vi "GDSIconEditor_CreateVIIcon.vi"(6 "ViRef(IgnoreIfNotWired)":refnum<vi>, 7 "AutomaticUpdateNoQuestionsAsked(False)":bool, 8 "error in (no error)":errorcluster, 9 "Application:Menu Launch:VI":string, 10 "Application:Menu Launch:App":refnum<vi>) -> (0 "error out":errorcluster)   [LabVIEW 2016]
uses:
  <resource>/Framework/Providers/Open_GDS/ClassProviders/Common/LvIcon_class/GDSLvIcon_ColorControl.ctl
  <resource>/Framework/Providers/Open_GDS/SubVIs/GOOP_HelpButton.ctl
  <resource>/Framework/Providers/Open_GDS/ClassProviders/Common/IconEditor/private/GDSIconEditor_ScopeType.ctl
  <vilib>/picture/picture.llb/imagedata.ctl
  <vilib>/Utility/miscctls.llb/LVPoint32TypeDef.ctl
  <resource>/Framework/Providers/Open_GDS/ClassProviders/Provider_LvNativeClass/ClassWriterNative_class/IconSize.ctl
  <resource>/Framework/Providers/Open_GDS/ClassProviders/Common/LvIcon_class/subvis/GDSLvIcon_TextDataType.ctl
  <resource>/Framework/Providers/Open_GDS/ClassProviders/Common/LvIcon_class/GDSLvIcon_WordCompressionType.ctl
  <resource>/Framework/Providers/Open_GDS/ClassProviders/Common/LvIcon_class/GDSLvIcon_TextAlignment.ctl
  <vilib>/Utility/miscctls.llb/LVRectTypeDef.ctl
  <vilib>/Utility/miscctls.llb/LVPositionTypeDef.ctl
  <vilib>/event_ctls.llb/lveventtype.ctl
  <vilib>/Utility/miscctls.llb/LVPointTypeDef.ctl
  <resource>/Framework/Providers/Open_GDS/ClassProviders/Provider_LvNativeClass/ClassWriterNative_class/ClassWriterNative.lvclass
  <vilib>/Utility/cursorutil.llb/Set Cursor (Icon Pict).vi
panel:
  in  "_HideHeader":bool=TRUE caption="Force Capital Letters"
  out "_IconPreview":picture caption="Icon Preview"
  out "DragIcon":picture
  in  "_MethodIconName":string caption="Body Text"
  in  "FloodFillMask":bool
  out "_IconName":string
  in  "_IconSearchText":string caption="Icon search text"
  in  "_Manage":bool
  in  "_Folders":u16(ring) caption="Folders" items=["<All icons>", "...EW 2014\\resource\\Framework\\Providers\\Icons", "...source\\Framework\\Providers\\Open_GDS\\Glyphs", "...esource\\Framework\\Providers\\Open_GDS\\Icons"]
  out "Icons":picture
  in  "_Icons":bool
  in  "_TextAlignment":u16(ring) caption="Text Alignment" items=["Center", "Left", "Right"]
  in  "_IconSize":u16(ring) caption="Icon Size" items=["Full", "1 c-term high", "2 c-term high", "3 c-term high", "4 c-term high"]
  in  "_HelpCreateViIcon":T1
  out "_FilePrefixFound":string caption="Prefix found"
  in  "_ApplyHeaderToAll":bool caption="Apply this header to all\nVIs/Ctrls in this folder"
  in  "_BodyTextColor":T2 caption="Body Text"
  in  "_BackgroundColor":T2 caption="Body Background"
  in  "_FontCompression":enum16{"Auto", "On", "Off"}(ring) caption="Font Compression"
  in  "_FontCapitalOnly":bool=TRUE caption="Force Capital Letters"
  out "_After":picture caption="New"
  out "_ViNotSavedMessage":string caption="VI not saved. Please select a path!"
  in  "Cancel":bool
  in  "Accept":bool
  in  "_EditHeader":bool
  in  "_TemplateVI":bool
  in  "_VIPath":path caption="VI Path"
  out "_Before":picture caption="Current"
  out "_Scope":string caption="Visibility"
  in  "Icon not available":picture
  in  "_OCR":bool
  # "Icon"
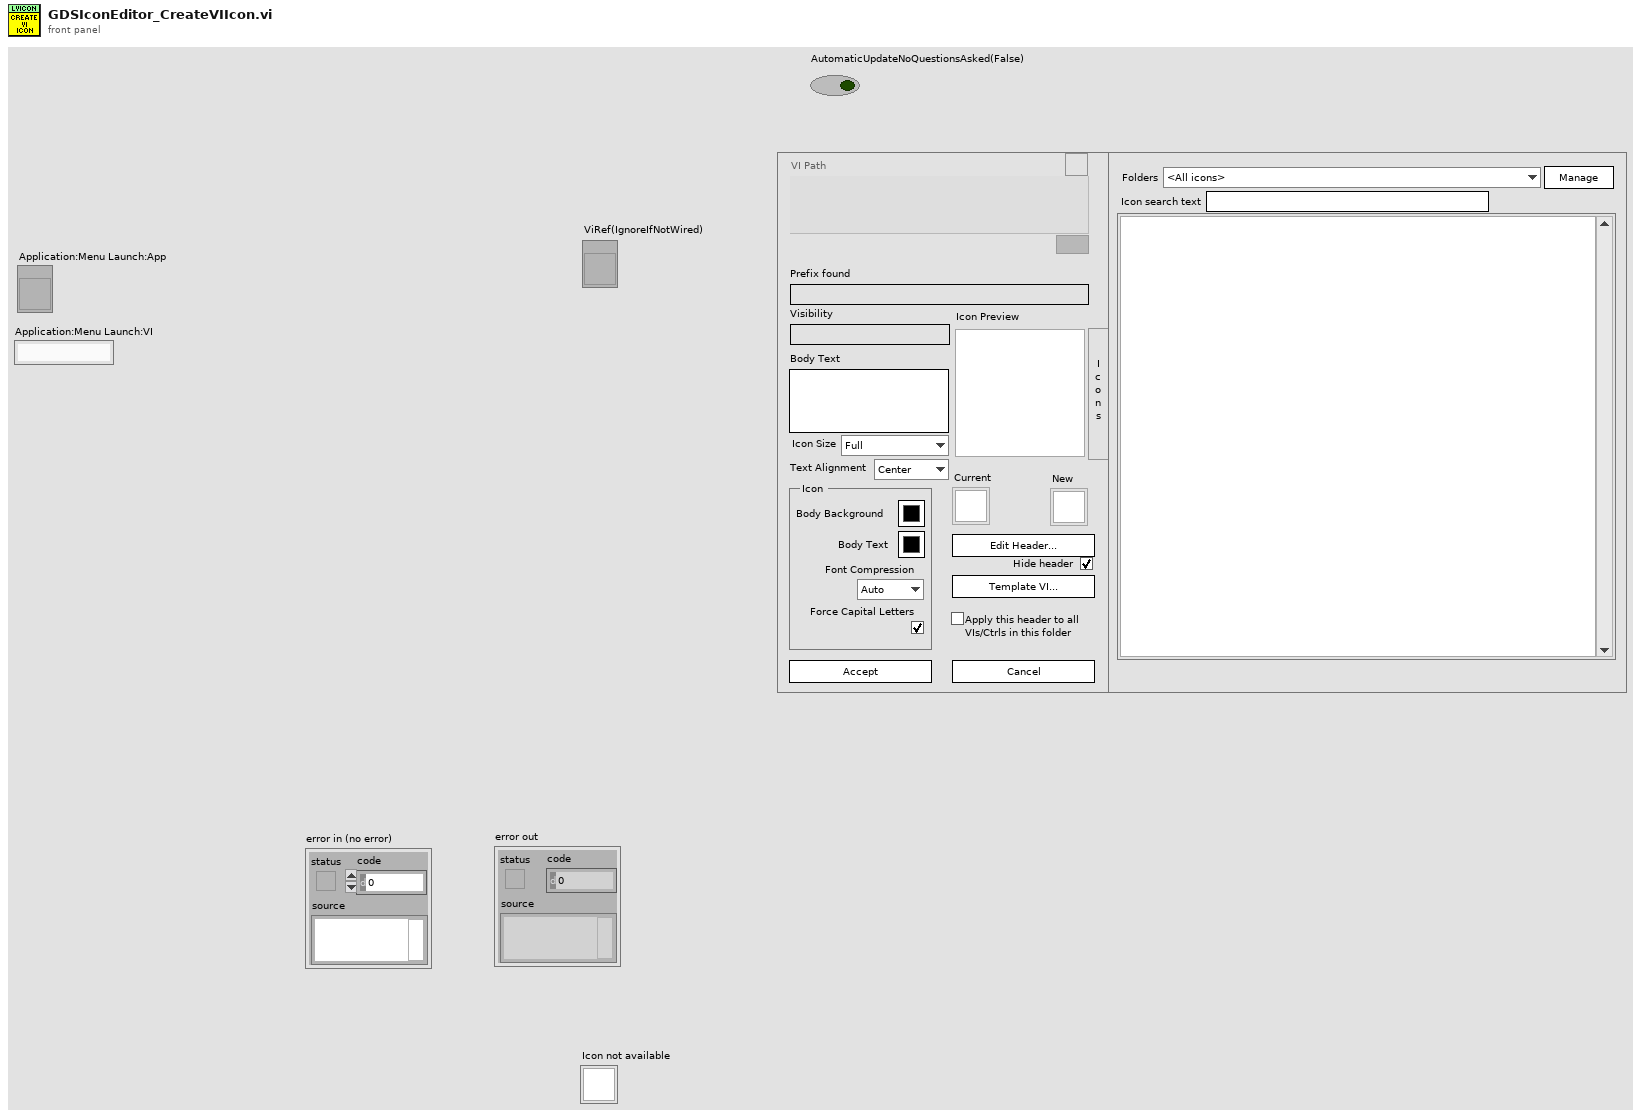
[diagram p1: front panel]
types:
  T1 = typedef "GOOP_HelpButton.ctl" = bool
  T2 = typedef "GDSLvIcon_ColorControl.ctl" = cluster{"Decal":bool, "Color":u32}
  T3 = typedef "GDSIconEditor_ScopeType.ctl" = enum16{"Public", "Proteced", "Private"}
  T4 = typedef "imagedata.ctl" = cluster{"image type":i32, "image depth":i32, "image":u8[], "mask":u8[], "colors":u32[], "Rectangle":cluster{"left":i16, "top":i16, "right":i16, "bottom":i16}}
  T5 = typedef "LVPoint32TypeDef.ctl" = cluster{"Horizontal":i32, "Vertical":i32}
  T6 = cluster{"License key":string, "Key info":string, "Prefix":string, "Header exists":bool, "Separator":string, "Folder":path, "VIs":path[], "VI Path":path, "VI exist":bool, "VI name":string, "Icon exist":bool, "ViRef":refnum<vi>, "LibraryRef":refnum<vi>, "Scope":T3, "FrameColor":u32, "Frame thickness":i32, "HeaderIcon":u8[][], "BodyIconHeight":i32, "BodyIconWidth":i32, "IconOut":u8[][], "AppRef":refnum<vi>, "Counter":i32, "Text1":string, "Text2":string, "Text0":string, "Type":enum16{"LvClass", "Library", "X-Control"}, "ConnectorPaneHeight":i32[], "StartRow":i32, "StartIconSize":u16, "Offset":cluster{"X":i32, "Y":i32}, "OldOffset":cluster{"X":i32, "Y":i32}, "Icons":T4[], "IconPos":cluster{"left":i16, "top":i16, "right":i16, "bottom":i16}[], "IconSelected":i32, "BgIcon":u8[][], "BgIconOffset":cluster{"X":i32, "Y":i32}, "Folders":path[], "DraggingIcon":bool, "BodyIcon":u8[][], "BgIconMask":u8[], "HeaderBkColor":u32, "CurrentIcon":cluster{"BgIcon":u8[][], "BgIconOffset":cluster{"X":i32, "Y":i32}, "BgIconMask":u8[], "ColorsOkayforiconToBeOnTopOf":u8[]}, "Moving":bool, "IconDropped":i32, "StartMethodName":string, "DraggingText":bool, "TextBounds":cluster{"FirstRow":i32, "FirstColumn":i32, "LastRow":i32, "LastColumn":i32}, "StartTextDraggingPos":T5, "NoControlsToMove":bool, "LayoutChangeExist":bool, "IconNames":string[], "IconPaths":cluster{i32, "path out":path}[], "Library":bool, "ClassBodyIcon":string, "FirstTime":bool, "TermWindowOpen":bool}
  T7 = typedef "LVBoundsTypeDef.ctl" = cluster{"Width":u32, "Height":u32}
  T8 = typedef "LVRectTypeDef.ctl" = cluster{"Left":i16, "Top":i16, "Right":i16, "Bottom":i16}
  T9 = typedef "ClassWriterNative.lvclass/IconSize.ctl" = enum16{"Full", "1 c-term high", "2 c-term high", "3 c-term high"}
  T10 = typedef "GDSLvIcon_TextDataType.ctl" = cluster{"Text":string, "Allow Only Capital Chars":bool, "Compression":T11, "Alignment":T12}
  T11 = typedef "GDSLvIcon_WordCompressionType.ctl" = enum16{"Auto", "On", "Off"}
  T12 = typedef "GDSLvIcon_TextAlignment.ctl" = enum16{"Center", "Left", "Right"}
  T13 = typedef "LVPositionTypeDef.ctl" = cluster{"Left":i32, "Top":i32}
  T14 = typedef "lveventtype.ctl" = enum32{"Null", "Timeout", "Annotation Menu Selection", "Annotation Menu Selection?", "App Instance Close", "App Instance Close?", "Autoscale Range Change", "Bookmark Info Change", "Cell Edit", "Cell Edit?", "Cursor Grab", "Cursor Grab?", "Cursor Menu Selection", "Cursor Menu Selection?", "Cursor Move", "Cursor Release", "Data Change", "Direction Change", "Display State Change", "Drag Ended", "Drag Enter", "Drag Leave", "Drag Over", "Drag Source Update", "Drag Starting", "Drag Starting?", "Drop", "Exec State Change", "Key Down", "Key Down?", "Key Repeat", "Key Repeat?", "Key Up", "Listbox Double Click", "Menu Activation?", "Menu Selection (App)", "Menu Selection? (App)", "Menu Selection (User)", "Mouse Down", "Mouse Down?", "Mouse Enter", "Mouse Leave", "Mouse Move", "Mouse Up", "Mouse Wheel", "NI Security User Change (App)", "Pane Size", "Panel Close", "Panel Close?", "Panel Resize", "Plot Attribute Change", "Scale Range Change", "Shortcut Menu Activation?", "Shortcut Menu Selection (App)", "Shortcut Menu Selection? (App)", "Shortcut Menu Selection (User)", "Tree Double Click", "Tree Drag", "Tree Drag?", "Tree Drop", "Tree Drop?", "Tree Item Close", "Tree Item Close?", "Tree Item Open", "Tree Item Open?", "User Event", "Value Change"}
  T15 = typedef "LVPointTypeDef.ctl" = cluster{"Horizontal":i16, "Vertical":i16}
  T16 = enum32{"invalid scope", "public", "private", "protected", "community"}
  T17 = typedef "Librarian File Info Out.ctl" = cluster{"creation date":u32, "last mod date":u32, "type":string, "creator":string, "LV version":i32, "size":i32, "top level":bool}
  T18 = enum32{"invalid VI type", "Standard VI", "Control VI", "Global VI", "Polymorphic VI", "Configuration VI", "SubSystem", "Facade VI", "Method VI", "Statechart Diagram VI"}
  T19 = typedef "GDSLvClass_IconSettingsType.ctl" = cluster{"Frame":u32, "Frame thickness":u8, "Header Background":u32, "Header Text":u32, "ColorPublic":u32, "ColorProtected":u32, "ColorPrivate":u32, "Body Text":u32, "ClassBodyIcon":string}
  T20 = cluster{"CtrlRef":refnum<vi>, "BeforeTerminalIndex":i32, "AfterTerminalIndex":i32}[]
  T21 = cluster{"BgIcon":u8[][], "BgIconOffset":cluster{"X":i32, "Y":i32}, "BgIconMask":u8[], "ColorsOkayforiconToBeOnTopOf":u8[]}
  T22 = cluster{"FirstRow":i32, "FirstColumn":i32, "LastRow":i32, "LastColumn":i32}
  T23 = typedef "eventvkey.ctl" = enum16{"ASCII", "Enter", "Return", "Shift", "Ctrl", "Alt", "Cmd", "Opt", "Caps", "NumLock", "Clear", "Break", "Up", "Down", "Left", "Right", "Insert", "Delete", "Home", "End", "PageUp", "PageDown", "Escape", "Help", "Pause", "ScrollLock", "F1", "F2", "F3", "F4", "F5", "F6", "F7", "F8", "F9", "F10", "F11", "F12", "F13", "F14", "F15", "F16", "F17", "F18", "F19", "F20", "F21", "F22", "F23", "F24", "Play", "VolumeUp", "VolumeDown", "Mute", "Two Byte Char"}
  T24 = cluster{"Shift":bool, "Ctrl":bool, "Alt":bool, "Cmd":bool, "Opt":bool}
  T25 = cluster{"left":i16, "top":i16, "right":i16, "bottom":i16}[]
  T26 = typedef "LVMouseTypeDef.ctl" = cluster{"Mouse Position":cluster{"X":i32, "Y":i32}, "Mouse Modifiers":cluster{"Button Down":bool, "Shift Mod":bool, "Menu Mod":bool, "Option Mod":bool}}
  T27 = typedef "ColorControl.ctl" = cluster{"Decal":bool, "Color":u32}
  T28 = cluster{"left":i16, "top":i16, "right":i16, "bottom":i16}
  T29 = enum32{"existing file", "new file", "new or existing file", "existing dir", "new dir", "new or existing dir", "existing file (use LLBs)", "new file (use LLBs)", "new or existing file (use LLBs)", "new or existing file or directory (use LLBs)", "existing dir (use LLBs)", "new dir (use LLBs)", "new or existing dir (use LLBs)", "existing file or dir", "new file or dir", "new or existing file or dir", "existing file or dir (use LLBs)", "new file or dir (use LLBs)"}
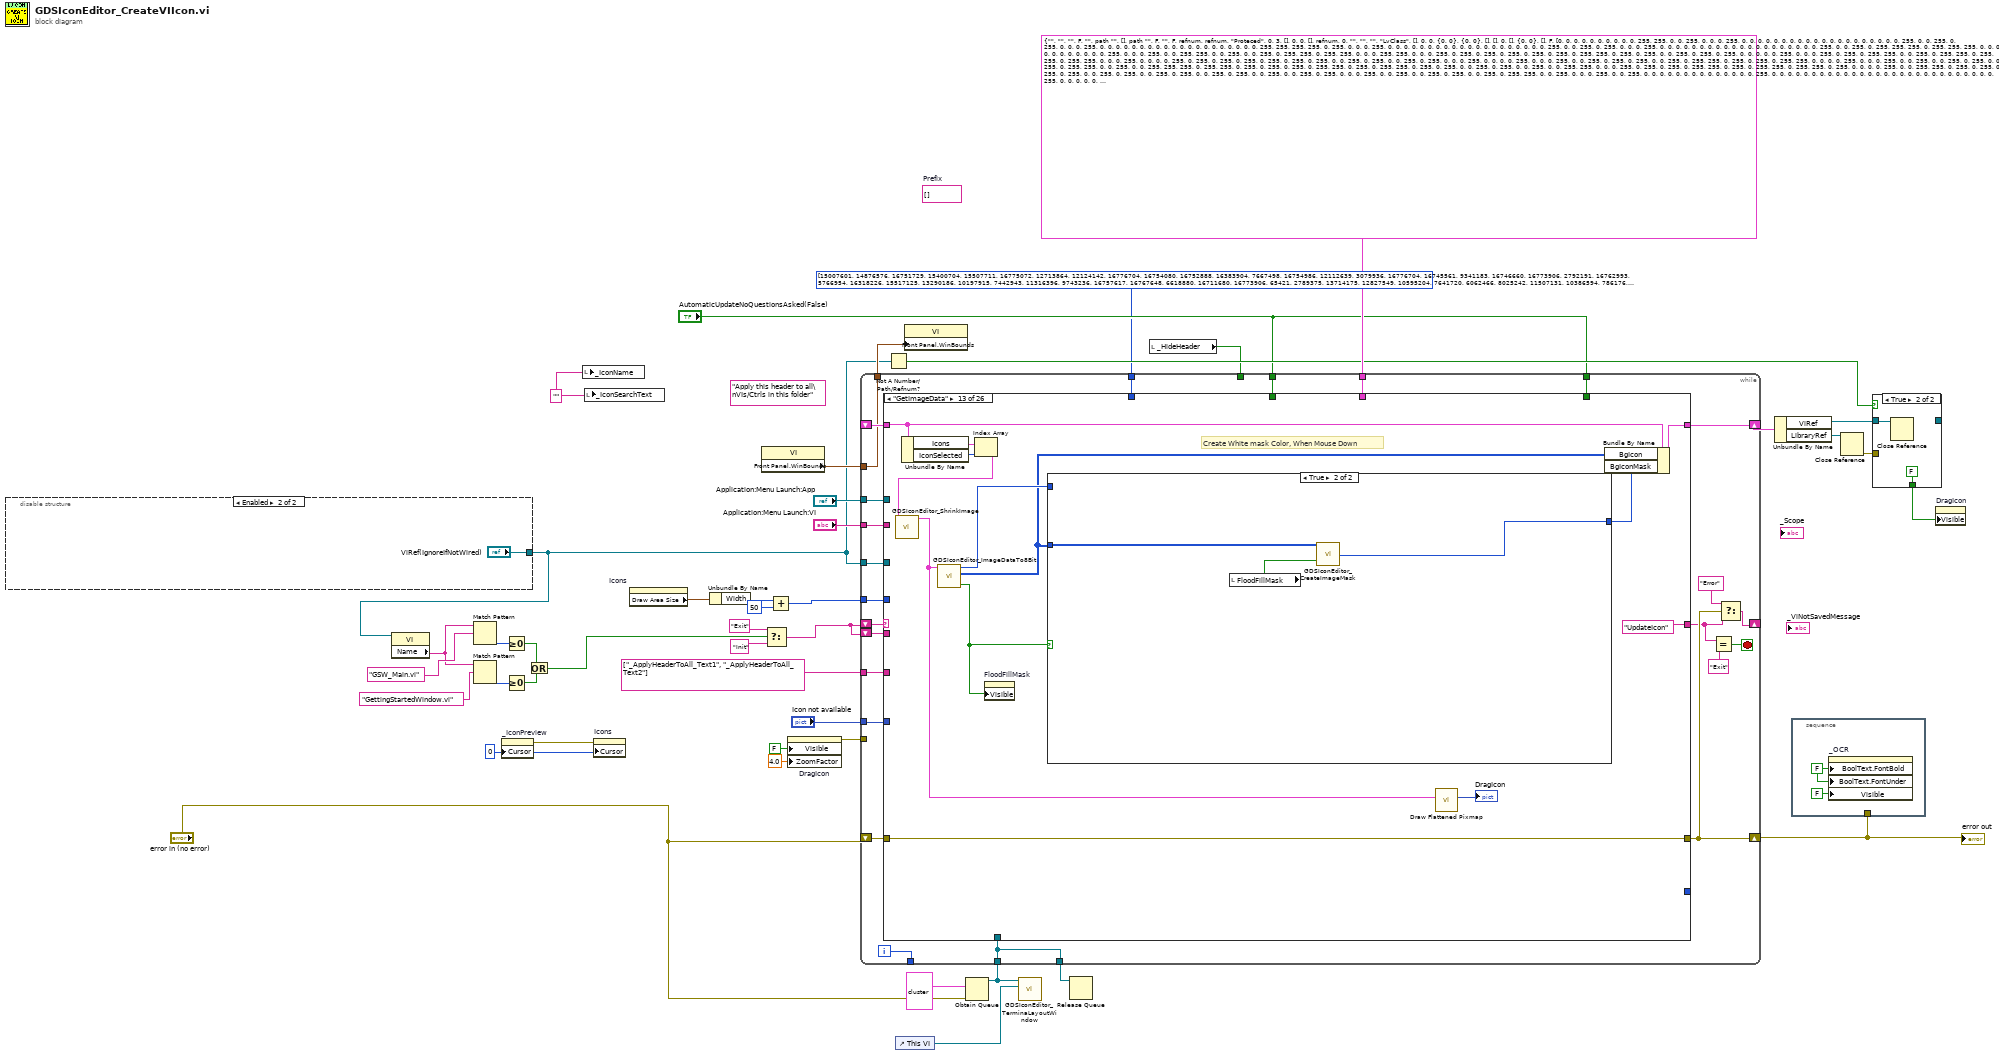
[diagram p0: block diagram]
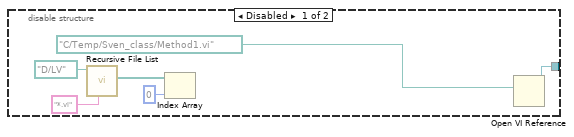
[diagram p2: hidden frame]
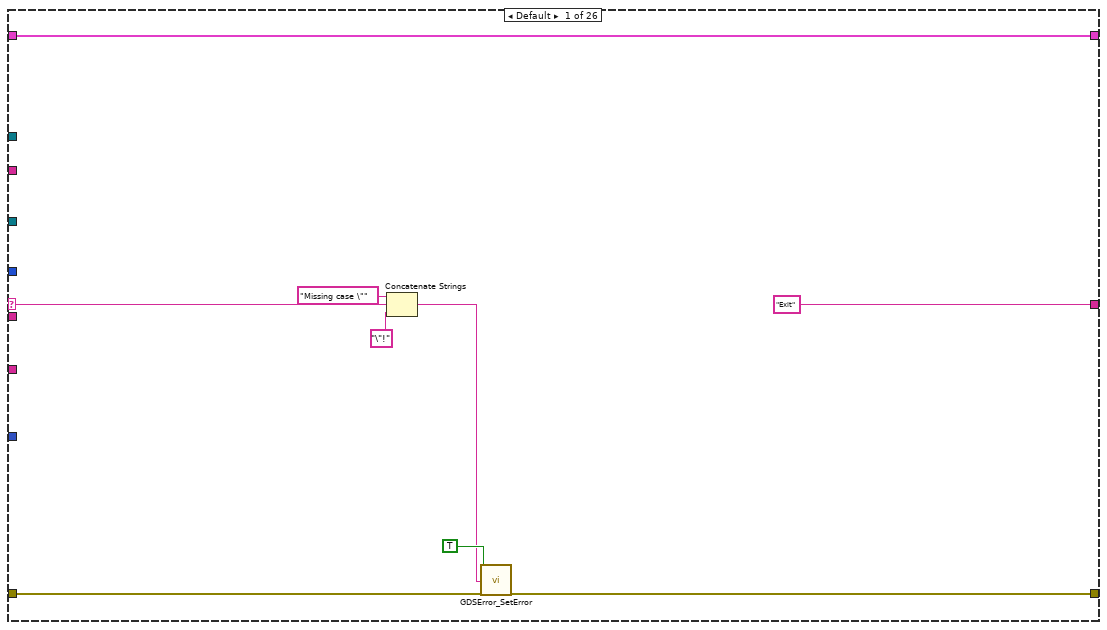
[diagram p4: hidden frame]
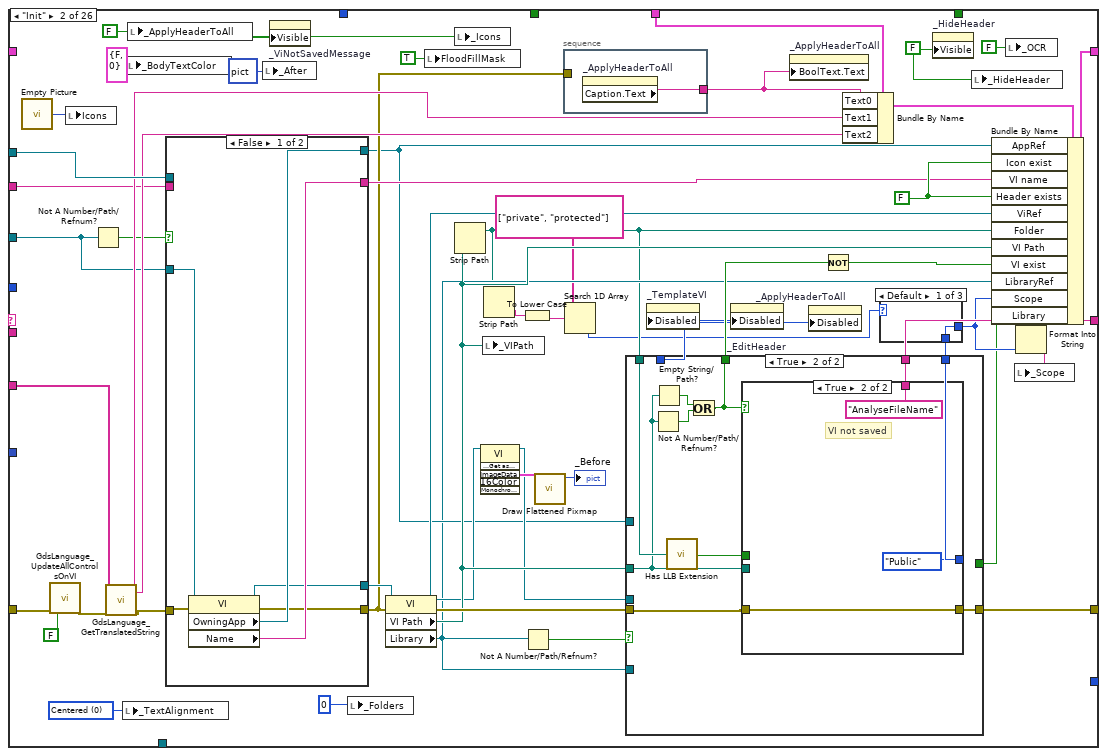
[diagram p5: hidden frame]
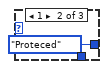
[diagram p6: hidden frame]
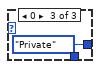
[diagram p7: hidden frame]
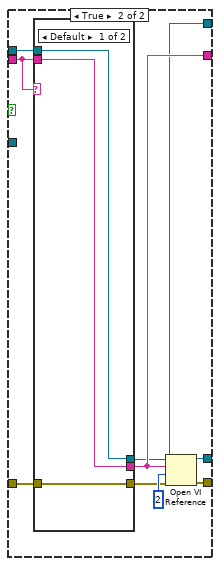
[diagram p8: hidden frame]
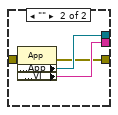
[diagram p9: hidden frame]
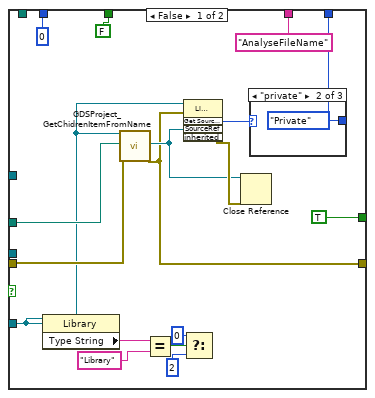
[diagram p10: hidden frame]
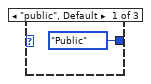
[diagram p11: hidden frame]
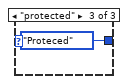
[diagram p12: hidden frame]
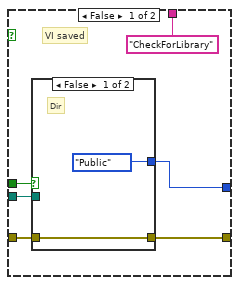
[diagram p13: hidden frame]
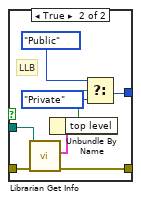
[diagram p14: hidden frame]
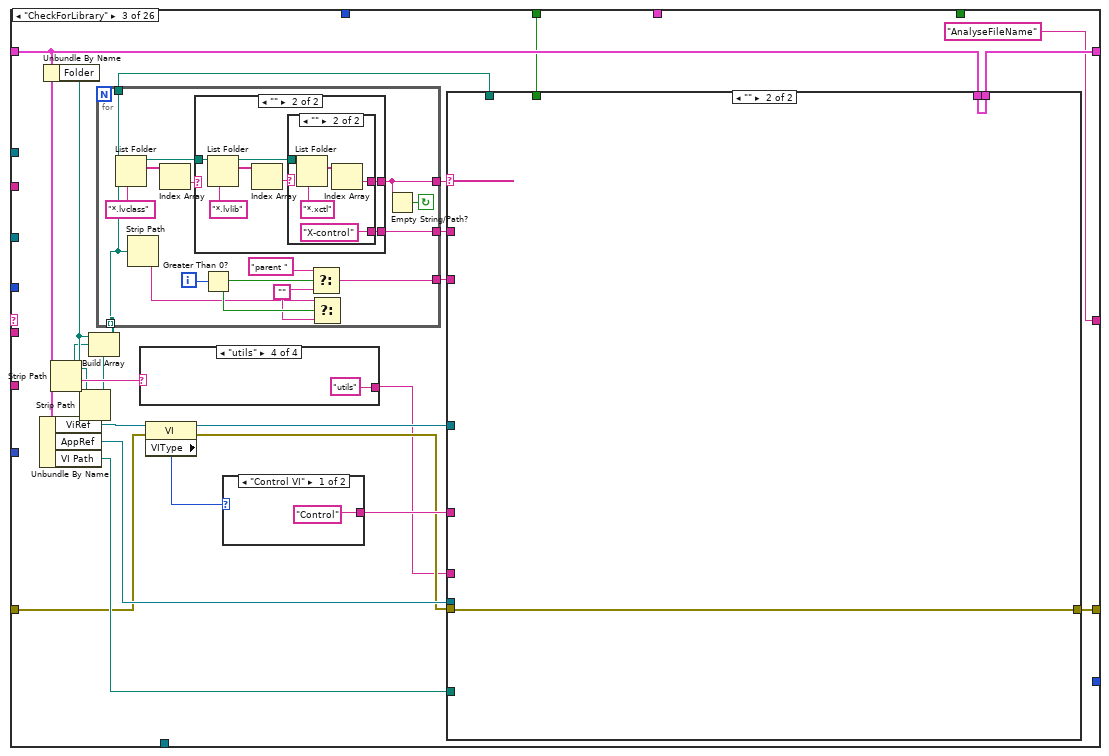
[diagram p15: hidden frame]
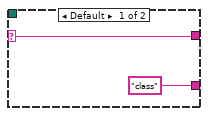
[diagram p16: hidden frame]
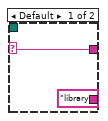
[diagram p17: hidden frame]
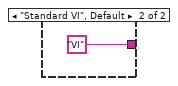
[diagram p18: hidden frame]
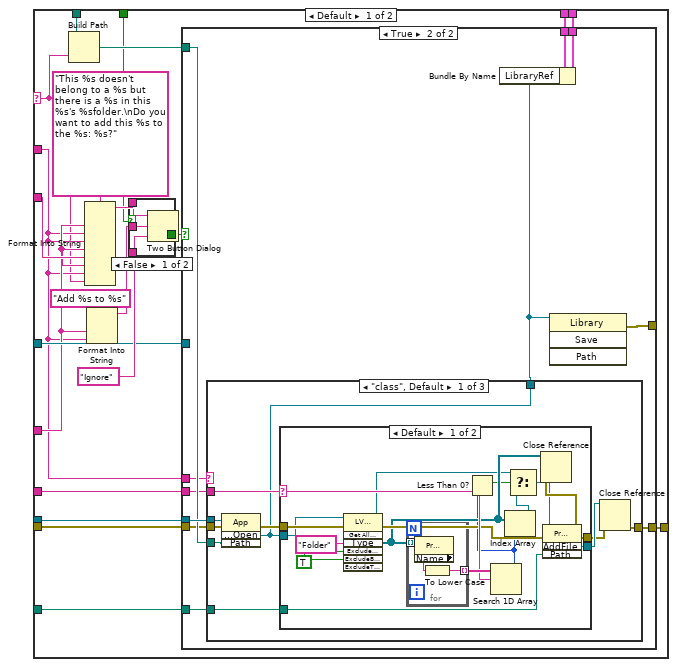
[diagram p19: hidden frame]
diagram:
  w18 = "" ("_IconSearchText")
  (unwired) string[] []  # Prefix
  w21 = 0 ("Cursor")
  (unwired) "Apply this header to all\nVIs/Ctrls in this folder" ("Caption.Text")
  n1 = disable-structure shown="Enabled" {
    disable-tunnel: [w50 "ViRef(IgnoreIfNotWired)"] -> w16
    frame Disabled {
      n2 = call <vilib>:"Recursive File List.vi"("pattern"="*.vi", "Folder Path"=path "D:/LV") -> ("All Files in Dir"=w47:path[])  [unwired: 5 in, 4 out]
      n3 = Index Array(array=w47, index=0) -> ()  [unwired: 1 out]
      n4 = Open VI Reference(vi path=path "C:/Temp/Sven_class/Method1.vi" ("Folder Path")) -> (vi reference=w50:refnum<vi>)  [unwired: 5 in, 1 out]
    }
    frame Enabled {
    }
  }
  n5 = property class="VI"(reference=w16) -> ("Name"=w5:string)  [unwired: 1 in, 2 out]
  n6 = Match Pattern(string=w5, regular expression="GSW_Main.vi" ("y")) -> (offset past match=w7:i32)  [unwired: 1 in, 3 out]
  n7 = Match Pattern(string=w5, regular expression="GettingStartedWindow.vi" ("y")) -> (offset past match=w6:i32)  [unwired: 1 in, 3 out]
  n8 = property on="_IconPreview" class="Pict"("Cursor"=w21) -> (error out=w20:errorcluster)  [unwired: 2 in, 1 out]
  n9 = Greater Or Equal To 0?(x=w7) -> (x >= 0?=w2:bool)
  n10 = Greater Or Equal To 0?(x=w6) -> (x >= 0?=w3:bool)
  n11 = Or(x=w2, y=w3) -> (x .or. y?=w12:bool)
  n12 = local write "_IconName"(w18) -> ()
  n13 = local write "_IconSearchText"(w18) -> ()
  n14 = property on="Icons" class="Pict"(error in=w20, "Cursor"=w21) -> ()  [unwired: 1 in, 2 out]
  n15 = property on="Icons" class="Pict"() -> ("Draw Area Size"=w27:T7)  [unwired: 2 in, 2 out]
  n16 = Unbundle By Name(w27) -> ("Width"=w29:u32)
  n17 = property class="VI"() -> ("Front Panel.WinBounds"=w19:T8)  [unwired: 2 in, 2 out]
  n18 = Select(t="Exit", s=w12, f="Init") -> (s? t:f=w13:string)
  n19 = Add(x=w29, y=u32 50) -> (x+y=w28:u32)
  n20 = property on="DragIcon" class="Pict"("Visible"=FALSE, "ZoomFactor"=sgl 4.0 ("Zoom Factor")) -> (error out=w24:errorcluster)  [unwired: 2 in, 1 out]
  n21 = Not A Number/Path/Refnum?(number/path/refnum=w16) -> (NaN/Path/Refnum?=w37:bool)
  n22 = control-ref of="This VI"() -> (w31:refnum<vi>)
  n23 = Obtain Queue(element data type=cluster{"Message":string, "Picture":picture} {"Message"="", "Picture"=bytes[0]} ("Message"), error in (no error)="error in (no error)") -> (queue out=w32:refnum<queue>)  [unwired: 3 in, 2 out]
  n24 = call <resource>:"GDSIconEditor_TerminaLayoutWindow.vi"("ViRef"=w31, "ControlQueue"=w32) -> ()  [unwired: 10 in]
  n25 = local read "_HideHeader"() -> (w1:bool)
  n26 = while {
    tunnel: "Icon not available" -> [w71]
    shift-left: "error in (no error)" -> [w74]
    shift-right: [w66] -> w17
    shift-left: _ -> [w72]
    shift-right: [w73] -> w43
    shift-left: w13 -> [w75]
    shift-right: [w65] -> _
    tunnel: "Application:Menu Launch:App" -> [w70]
    tunnel: "Application:Menu Launch:VI" -> [w69]
    tunnel: T6 {"License key"="", "Key info"="", "Prefix"="", "Header exists"=FALSE, "Separator"="", "Folder"=path "", "VIs"=[], "VI Path"=path "", "VI exist"=FALSE, "VI name"="", "Icon exist"=FALSE, "ViRef"=refnum, "LibraryRef"=refnum, "Scope"=enum."Proteced", "FrameColor"=0, "Frame thickness"=3, "HeaderIcon"=[], "BodyIconHeight"=0, "BodyIconWidth"=0, "IconOut"=[], "AppRef"=refnum, "Counter"=0, "Text1"="", "Text2"="", "Text0"="", "Type"=enum."LvClass", "ConnectorPaneHeight"=[], "StartRow"=0, "StartIconSize"=0, "Offset"={"X"=0, "Y"=0}, "OldOffset"={"X"=0, "Y"=0}, "Icons"=[], "IconPos"=[], "IconSelected"=0, "BgIcon"=[], "BgIconOffset"={"X"=0, "Y"=0}, "Folders"=[], "DraggingIcon"=FALSE, "BodyIcon"=[[0, 0, 0, 0, 0, 0, 0, 0, 0, 0, 255, 255, 0, 0, 255, 0, 0, 0, 255, 0, 0, 0, 0, 0, 0, 0, 0, 0, 0, 0], [0, 0, 0, 0, 0, 0, 0, 0, 0, 255, 0, 0, 255, 0, 255, 0, 0, 0, 255, 0, 0, 0, 0, 0, 0, 0, 0, 0, 0, 0], [0, 0, 0, 0, 0, 0, 0, 0, 0, 255, 255, 255, 255, 0, 255, 0, 0, 0, 255, 0, 0, 0, 0, 0, 0, 0, 0, 0, 0, 0], [0, 0, 0, 0, 0, 0, 0, 0, 0, 255, 0, 0, 255, 0, 255, 0, 0, 0, 255, 0, 0, 0, 0, 0, 0, 0, 0, 0, 0, 0], [0, 0, 0, 0, 0, 0, 0, 0, 0, 255, 0, 0, 255, 0, 255, 255, 255, 0, 255, 255, 255, 0, 0, 0, 0, 0, 0, 0, 0, 0], [0, 0, 255, 0, 0, 0, 255, 0, 0, 255, 255, 0, 0, 255, 0, 0, 255, 0, 255, 255, 0, 255, 255, 0, 0, 0, 255, 255, 0, 0], [0, 255, 0, 255, 0, 255, 0, 255, 0, 255, 0, 255, 0, 255, 255, 0, 255, 0, 255, 0, 0, 255, 0, 255, 0, 255, 0, 0, 0, 0], [0, 255, 0, 0, 0, 255, 0, 255, 0, 255, 255, 0, 0, 255, 0, 255, 255, 0, 255, 255, 0, 255, 255, 0, 0, 0, 255, 0, 0, 0], [0, 255, 0, 255, 0, 255, 0, 255, 0, 255, 0, 255, 0, 255, 0, 0, 255, 0, 255, 0, 0, 255, 0, 255, 0, 0, 0, 255, 0, 0], [0, 0, 255, 0, 0, 0, 255, 0, 0, 255, 0, 255, 0, 255, 0, 0, 255, 0, 255, 255, 0, 255, 0, 255, 0, 255, 255, 0, 0, 0], [0, 255, 0, 0, 0, 255, 0, 0, 255, 0, 0, 255, 0, 255, 0, 0, 255, 0, 255, 255, 0, 0, 255, 0, 0, 255, 255, 255, 0, 255], [255, 0, 255, 0, 255, 0, 255, 0, 255, 255, 0, 255, 0, 255, 255, 0, 255, 0, 255, 0, 0, 255, 0, 255, 0, 0, 255, 0, 0, 255], [255, 0, 0, 0, 255, 0, 255, 0, 255, 0, 255, 255, 0, 255, 0, 255, 255, 0, 255, 255, 0, 255, 0, 0, 0, 0, 255, 0, 0, 255], [255, 0, 255, 0, 255, 0, 255, 0, 255, 0, 0, 255, 0, 255, 0, 0, 255, 0, 255, 0, 0, 255, 0, 255, 0, 0, 255, 0, 0, 255], [0, 255, 0, 0, 0, 255, 0, 0, 255, 0, 0, 255, 0, 255, 0, 0, 255, 0, 255, 255, 0, 0, 255, 0, 0, 0, 255, 0, 0, 255], [0, 0, 0, 0, 0, 0, 0, 0, 0, 0, 0, 0, 0, 0, 255, 0, 0, 0, 0, 0, 0, 0, 0, 0, 0, 0, 0, 0, 0, 0], [0, 0, 0, 0, 0, 0, 0, 0, 0, 0, 0, 0, 0, 255, 0, 0, 0, 0, 0, 0, 0, 0, 0, 0, 0, 0, 0, 0, 0, 0], [0, 0, 0, 0, 0, 0, 0, 0, 0, 0, 0, 0, 0, 255, 255, 0, 0, 0, 0, 0, 0, 0, 0, 0, 0, 0, 0, 0, 0, 0], [0, 0, 0, 0, 0, 0, 0, 0, 0, 0, 0, 0, 0, 255, 0, 255, 0, 0, 0, 0, 0, 0, 0, 0, 0, 0, 0, 0, 0, 0], [0, 0, 0, 0, 0, 0, 0, 0, 0, 0, 0, 0, 0, 0, 255, 0, 0, 0, 0, 0, 0, 0, 0, 0, 0, 0, 0, 0, 0, 0], [0, 0, 0, 0, 0, 0, 0, 0, 0, 0, 0, 0, 0, 0, 0, 0, 0, 0, 0, 0, 0, 0, 0, 0, 0, 0, 0, 0, 0, 0], [0, 0, 0, 0, 0, 0, 0, 0, 0, 0, 0, 0, 0, 0, 0, 0, 0, 0, 0, 0, 0, 0, 0, 0, 0, 0, 0, 0, 0, 0]], "BgIconMask"=[], "HeaderBkColor"=0, "CurrentIcon"={"BgIcon"=[], "BgIconOffset"={"X"=0, "Y"=0}, "BgIconMask"=[], "ColorsOkayforiconToBeOnTopOf"=[]}, "Moving"=FALSE, "IconDropped"=-1, "StartMethodName"="", "DraggingText"=FALSE, "TextBounds"={"FirstRow"=2, "FirstColumn"=1, "LastRow"=6, "LastColumn"=27}, "StartTextDraggingPos"={"Horizontal"=0, "Vertical"=0}, "NoControlsToMove"=FALSE, "LayoutChangeExist"=FALSE, "IconNames"=[], "IconPaths"=[], "Library"=FALSE, "ClassBodyIcon"="", "FirstTime"=TRUE, "TermWindowOpen"=FALSE} ("Local data") -> [w62]
    shift-left: w13 -> [w61]
    tunnel: string[] ["_ApplyHeaderToAll_Text1", "_ApplyHeaderToAll_Text2"] -> [w60]
    tunnel: w16 -> [w59]
    tunnel: w32 -> [w58]
    tunnel: [w58] -> w33
    tunnel: w28 -> [w57]
    tunnel: w19 -> [w56]
    tunnel: [w56] -> w26
    tunnel: w24 -> [_]
    tunnel: [w55] -> _
    tunnel: "AutomaticUpdateNoQuestionsAsked(False)" -> [w54]
    tunnel: "AutomaticUpdateNoQuestionsAsked(False)" -> [w53]
    tunnel: u32[] [15007601, 14876576, 16751729, 15400704, 15507711, 16775072, 12713864, 12124142, 16776704, 16754080, 16752888, 16383904, 7667498, 16754986, 12112639, 3079936, 16776704, 16745561, 9341183, 16746660, 16773906, 2792191, 16762993, 5766954, 16318226, 15517125, 13290186, 10197915, 7442943, 11316396, 9743236, 16757617, 16767648, 6618880, 16711680, 16773906, 65421, 2789375, 13714175, 12827549, 10595204, 7641720, 6062466, 8025242, 11507131, 10386594, 786176, 8584960, 16318208, 16731648, 16755616, 16734715, 14399157, 16754801, 16714752, 10026888, 3524608] -> [w52]
    tunnel: w1 -> [_]
    i -> [w55]
    stop <- w68 stop-if-true
    n27 = case shown="\"GetImageData\"" w75 {
      selector: w75 -> [w77 _ _ _ _ _ w781 _ _ w903 _ _ _ w1450 _ _ _ w1631 _ _ _ _ _ _ _ _]
      tunnel: ["Exit" w102 "AnalyseFileName" "Auto find header" "DoIconTextOCR" "DoIconTextOCR_Before" ("t") w776 "Generate icon" "ShowLayoutChange" ("item tag") w939 w963 w1035 "UpdateIcon" ("y") w1457 "ReadIcons" "Generate icon" "DrawIcons" ("y") "Idle" ("y") "Idle" ("y") "Exit" w1784 w1832 w1894 "Exit" ("y") w1956 "Exit" ("y")] -> w64
      tunnel: w74 -> [w84 w117 w220 w410 w520 w727 w785 w800 w834 w902 w981 w1036 w1431 w1485 w1517 w1582 w1593 w1641 w1766 w1777 w1796 w1841 w1902 w1926 w1958 w2003]
      tunnel: [w83 w131 w219 w417 w521 w753 w786 w799 w833 w899 w980 w1036 w1431 w1485 w1516 w1582 w1588 w1643 w1766 w1774 w1797 w1842 w1887 w1925 w1957 w2003] -> w66
      tunnel: [w80 w135 w233 w416 w507 w754 w773 w797 w830 w906 w966 w1021 w1433 w1454 w1526 w1583 w1598 w1656 w1762 w1778 w1799 w1844 w1890 w1930 w1953 w2002] -> w73
      tunnel: w72 -> [w80 _ w229 w409 w516 w752 w774 w798 w831 w907 w967 w1022 w1434 w1454 w1527 w1584 w1596 w1644 w1769 w1778 w1798 w1843 w1890 w1930 w1954 w2002]
      tunnel: w71 -> [_ _ _ _ _ _ _ _ _ _ _ _ _ _ _ _ _ _ _ _ _ _ _ _ _ _]
      tunnel: w70 -> [_ w127 _ _ _ _ _ _ _ _ _ _ _ _ _ _ _ _ _ _ _ _ _ _ _ _]
      tunnel: w69 -> [_ w108 _ _ _ _ _ _ _ _ _ _ _ _ _ _ _ _ _ _ _ _ _ _ _ _]
      tunnel: w62 -> [_ w110 _ _ _ _ _ _ _ _ _ _ _ _ _ _ _ _ _ _ _ _ _ _ _ _]
      tunnel: w61 -> [_ _ _ _ _ _ _ _ _ _ _ _ _ _ _ _ _ _ _ _ _ _ _ _ _ w2004]
      tunnel: w60 -> [_ w114 _ _ _ _ _ _ _ _ _ _ _ _ _ _ _ _ _ _ _ _ _ _ _ _]
      tunnel: w59 -> [_ w103 _ _ _ _ _ _ _ _ _ _ _ _ _ _ _ _ _ _ _ _ _ _ _ _]
      tunnel: w58 -> [_ _ _ _ _ _ _ _ _ _ w979 w1010 _ _ _ _ _ _ _ _ _ _ _ _ _ _]
      tunnel: w57 -> [_ _ _ _ _ _ _ _ _ _ _ w1011 _ _ _ _ _ _ _ _ _ _ _ _ _ _]
      tunnel: [_ _ _ _ _ _ _ _ _ w896 _ _ _ _ _ _ _ _ _ _ _ _ _ _ _ _] -> _
      tunnel: w54 -> [_ _ w211 _ _ _ _ _ _ _ _ _ _ _ _ _ _ _ _ _ _ _ _ _ _ _]
      tunnel: w53 -> [_ _ _ _ _ _ _ _ _ w895 w962 _ _ _ _ _ _ _ _ _ _ _ _ _ _ _]
      tunnel: w52 -> [_ _ _ _ w505 w720 _ _ _ _ _ _ _ _ _ _ _ _ _ _ _ _ _ _ _ _]
      frame Default {
        n28 = Concatenate Strings("Missing case \"" ("source"), w77, "\"!") -> (w76:string)
        n29 = call <resource>:"GDSError_SetError.vi"("status"=TRUE, "source"=w76, "error in (no error)"=w84) -> ("error out"=w83:errorcluster)  [unwired: 16 in]
      }
      frame "Init" {
        w85 = FALSE ("_OCR")
        w99 = u16 0 items=["Centered", "Left", "Right"] ("_TextAlignment")
        w97 = FALSE ("ApplyToAll")
        w130 = FALSE ("Header exists")
        n30 = call "Empty Picture"() -> ("empty picture"=w96:picture)
        n31 = call <resource>:"GdsLanguage_UpdateAllControlsOnVI.vi"("error in (no error)"=w117, "CreateLanguageFile(Use this to create a languageFile)"=FALSE) -> ("error out"=w115:errorcluster)  [unwired: 16 in, 1 out]
        n32 = local write "Icons"(w96) -> ()
        n33 = Not A Number/Path/Refnum?(number/path/refnum=w103) -> (NaN/Path/Refnum?=w105:bool)
        n34 = call <resource>:"GdsLanguage_GetTranslatedString.vi"("StringID(s)"=w114, "error in (no error)"=w115) -> ("FirstStringOut"=w112:string, "SecondStringOut"=w111:string, "error out"=w109:errorcluster)  [unwired: 14 in, 1 out]
        n35 = local write "_TextAlignment"(w99) -> ()
        n36 = local write "_BodyTextColor"(T2 {"Decal"=FALSE, "Color"=0} ("BodyText")) -> ()
        n37 = local write "_ApplyHeaderToAll"(w97) -> ()
        n38 = case shown="False" w105 {
          tunnel: [w140 w152] -> w134
          tunnel: [w141 w151] -> w129
          tunnel: w127 -> [_ w149]
          tunnel: [w142 w148] -> w104
          tunnel: w109 -> [w144 w147]
          tunnel: w108 -> [_ w146]
          tunnel: [w139 w145] -> w107
          tunnel: w103 -> [w143 _]
          frame False {
            n39 = property class="VI"(reference=w143, error in=w144) -> (reference out=w140:refnum<vi>, error out=w139:errorcluster, "OwningApp"=w142:refnum<vi>, "Name"=w141:string)
          }
          frame True {
            n40 = case shown="Default" w146 {
              tunnel: [w156 w160] -> w148
              tunnel: [w155 w159] -> w151
              tunnel: [w154 w158] -> w150
              tunnel: w147 -> [w154 w157]
              tunnel: w149 -> [w156 _]
              tunnel: w146 -> [w155 _]
              frame Default {
              }
              frame "" {
                n41 = property class="App"(error in=w157) -> (error out=w158:errorcluster, "Application:Menu Launch:App"=w160:refnum<vi>, "Application:Menu Launch:VI"=w159:string)  [unwired: 1 in, 1 out]
              }
            }
            n42 = Open VI Reference(application reference (local)=w148, vi path=w151, options=2, error in (no error)=w150) -> (vi reference=w152:refnum<vi>, error out=w145:errorcluster)  [unwired: 2 in]
          }
        }
        n43 = local write "_After"(picture bytes[1054] ("After")) -> ()
        n44 = property on="_ViNotSavedMessage" class="Str"("Visible"=w97) -> ()  [unwired: 2 in, 2 out]
        n45 = local write "_Folders"(0) -> ()
        n46 = property class="VI"(reference=w134, error in=w107) -> (reference out=w121:refnum<vi>, error out=w128:errorcluster, "VI Path"=w126:path, "Library"=w101:refnum<vi>)
        n47 = local write "FloodFillMask"(TRUE ("FloodFillMask")) -> ()
        n48 = local write "_Icons"(w97) -> ()
        n49 = Strip Path(path=w126) -> (stripped path=w93:path)  [unwired: 1 out]
        n50 = invoke class="VI" method="VI Icon.Get as Image Data"(reference=w121) -> (reference out=w120:refnum<vi>, "ImageData"=w123:T4)  [unwired: 5 in, 4 out]
        n51 = local write "_VIPath"(w126) -> ()
        n52 = Strip Path(path=w93) -> (name=w92:string)  [unwired: 1 out]
        n53 = To Lower Case(string=w92) -> (all lower case string=w95:string)
        n54 = Not A Number/Path/Refnum?(number/path/refnum=w101) -> (NaN/Path/Refnum?=w100:bool)
        n55 = call <vilib>:"Draw Flattened Pixmap.vi"("image data"=w123) -> ("new picture"=→"_Before":picture)  [unwired: 8 in]
        n56 = stacked-sequence {
          tunnel: [w161] -> w106
          tunnel: w107 -> [_]
          frame #0 {
            n57 = property on="_ApplyHeaderToAll" class="Bool (strict)"() -> ("Caption.Text"=w161:string)  [unwired: 2 in, 2 out]
          }
        }
        n58 = Search 1D Array(1D array=string[] ["private", "protected"], element=w95) -> (index of element=w91:i32)  [unwired: 1 in]
        n59 = case shown="True" w100 {
          tunnel: [FALSE ("Cleared?") w184] -> w132
          tunnel: [w171 w191] -> w131
          tunnel: [w174 w189] -> w90
          tunnel: w93 -> [_ w185]
          tunnel: w128 -> [w176 w188]
          tunnel: w126 -> [w177 w183]
          tunnel: w120 -> [_ _]
          tunnel: w101 -> [w169 _]
          tunnel: [u8 0 ("t") _] -> w118
          tunnel: w104 -> [_ _]
          tunnel: ["AnalyseFileName" w182] -> w102
          tunnel: [TRUE ("Cleared?") _] -> w88
          frame False {
            n60 = property class="Library"(reference=w169) -> ("Type String"=w168:string)  [unwired: 1 in, 2 out]
            n61 = call <resource>:"GDSProject_GetChidrenItemFromName.vi"("ProjectItemToSearchFrom"=w169, "ItemToSearchForInProjectTreeBasedOnPath(used if wired)"=w177, "error in (no error)"=w176) -> ("ProjectItemFound"=w172:refnum<vi>, "error out"=w171:errorcluster)  [unwired: 13 in, 2 out]
            n62 = Equal?(x=w168, y="Library") -> (x = y?=w166:bool)
            n63 = invoke class="Library" method="Get Source Scope"(reference=w169, error in=w171, "SourceRef"=w172) -> (error out=w173:errorcluster, "GetSourceScope"=w175:T16)  [unwired: 2 in, 3 out]
            n64 = Select(t=u8 0, s=w166, f=u8 2 ("Disabled")) -> ()  [unwired: 1 out]
            n65 = Close Reference(reference=w172, error in (no error)=w173) -> ()  [unwired: 1 out]
            n66 = case shown="\"private\"" w175 {
              tunnel: [GDSIconEditor_ScopeType."Public" ("Scope") GDSIconEditor_ScopeType."Private" ("Scope") GDSIconEditor_ScopeType."Proteced" ("Scope")] -> w174
              frame "public", Default {
              }
              frame "private" {
              }
              frame "protected" {
              }
            }
          }
          frame True {
            n67 = Not A Number/Path/Refnum?(number/path/refnum=w183) -> (NaN/Path/Refnum?=w186:bool)
            n68 = Empty String/Path?(string/path=w183) -> (empty?=w187:bool)
            n69 = call <vilib>:"Has LLB Extension.vi"("path"=w185) -> ("path to VI library?"=w190:bool)
            n70 = Or(x=w187, y=w186) -> (x .or. y?=w184:bool)
            n71 = case shown="True" w184 {
              tunnel: w188 -> [w197 w210]
              tunnel: [w193 w210] -> w191
              tunnel: w183 -> [w196 _]
              tunnel: w190 -> [w195 _]
              tunnel: [w194 GDSIconEditor_ScopeType."Public" ("Scope")] -> w189
              tunnel: ["CheckForLibrary" "AnalyseFileName"] -> w182
              frame False {
                # "VI saved"
                n72 = case shown="False" w195 {
                  tunnel: w197 -> [w199 w207]
                  tunnel: [w199 w206] -> w193
                  tunnel: w196 -> [_ w205]
                  tunnel: [GDSIconEditor_ScopeType."Public" ("Scope") w203] -> w194
                  frame False {
                    # "Dir"
                  }
                  frame True {
                    # "LLB"
                    n73 = call <vilib>:"Librarian Get Info.vi"("error in (no error)"=w207, "path"=w205) -> ("error out"=w206:errorcluster, "file information"=w204:T17)  [unwired: 7 in, 1 out]
                    n74 = Unbundle By Name(w204) -> ("top level"=w202:bool)
                    n75 = Select(t=GDSIconEditor_ScopeType."Public" ("Scope"), s=w202, f=GDSIconEditor_ScopeType."Private" ("Scope")) -> (s? t:f=w203:T3)
                  }
                }
              }
              frame True {
                # "VI not saved"
              }
            }
          }
        }
        n76 = property on="_TemplateVI" class="Bool"("Disabled"=w118) -> ()  [unwired: 2 in, 2 out]
        n77 = property on="_EditHeader" class="Bool"("Disabled"=w118) -> ()  [unwired: 2 in, 2 out]
        n78 = property on="_ApplyHeaderToAll" class="Bool (strict)"("BoolText.Text"=w106) -> ()  [unwired: 2 in, 2 out]
        n79 = property on="_ApplyHeaderToAll" class="Bool (strict)"("Disabled"=w118) -> ()  [unwired: 2 in, 2 out]
        n80 = Not(x=w132) -> (.not. x?=w133:bool)
        n81 = Bundle By Name(cluster=w110, "Text0"=w106, "Text1"=w112, "Text2"=w111) -> (w113:T6)
        n82 = case shown="Default" w91 {
          tunnel: w90 -> [w136 _ _]
          tunnel: [w136 GDSIconEditor_ScopeType."Proteced" ("Scope") GDSIconEditor_ScopeType."Private" ("Scope")] -> w89
          frame Default {
          }
          frame 1 {
          }
          frame 0 {
          }
        }
        n83 = property on="_HideHeader" class="Bool (strict)"("Visible"=w85) -> ()  [unwired: 2 in, 2 out]
        n84 = local write "_HideHeader"(w85) -> ()
        n85 = Bundle By Name(cluster=w113, "AppRef"=w104, "Icon exist"=w130, "VI name"=w129, "Header exists"=w130, "ViRef"=w121, "Folder"=w93, "VI Path"=w126, "VI exist"=w133, "LibraryRef"=w101, "Scope"=w89, "Library"=w88) -> (w135:T6)
        n86 = local write "_OCR"(FALSE ("_OCR")) -> ()
        n87 = Format Into String(w89) -> (resulting string=w125:string)  [unwired: 3 in, 1 out]
        n88 = local write "_Scope"(w125) -> ()
      }
      frame "CheckForLibrary" {
        n89 = Unbundle By Name(w229) -> ("ViRef"=w228:refnum<vi>, "AppRef"=w223:refnum<vi>, "VI Path"=w222:path)
        n90 = Unbundle By Name(w229) -> ("Folder"=w217:path)
        n91 = Strip Path(path=w217) -> (stripped path=w213:path, name=w231:string)
        n92 = Strip Path(path=w213) -> (stripped path=w212:path)  [unwired: 1 out]
        n93 = Build Array(w217, w213, w212) -> (w216:path[])
        n94 = for {
          tunnel: [w241] -> w230
          tunnel: [w243] -> w225
          tunnel: w216 -> [w242] mode=indexing
          tunnel: [w242] -> w215
          tunnel: [w237] -> w214
          i -> [w239]
          stop <- w240 continue-if-true
          w235 = ""
          n95 = List Folder(path=w242, pattern="*.lvclass") -> (path out=w244:path, filenames=w246:string[])  [unwired: 2 in, 2 out]
          n96 = Strip Path(path=w242) -> (name=w234:string)  [unwired: 1 out]
          n97 = Index Array(array=w246) -> (element=w245:string)  [unwired: 1 in]
          n98 = case shown="\"\"" w245 {
            selector: w245 -> [w249 _]
            tunnel: w244 -> [_ w254]
            tunnel: [w249 w251] -> w241
            tunnel: ["class" ("pattern") w250] -> w243
            frame Default {
            }
            frame "" {
              n99 = List Folder(path=w254, pattern="*.lvlib") -> (path out=w252:path, filenames=w256:string[])  [unwired: 2 in, 2 out]
              n100 = Index Array(array=w256) -> (element=w253:string)  [unwired: 1 in]
              n101 = case shown="\"\"" w253 {
                selector: w253 -> [w258 _]
                tunnel: w252 -> [_ w261]
                tunnel: [w258 w260] -> w251
                tunnel: ["library" ("pattern") "X-control" ("pattern")] -> w250
                frame Default {
                }
                frame "" {
                  n102 = List Folder(path=w261, pattern="*.xctl") -> (filenames=w262:string[])  [unwired: 2 in, 3 out]
                  n103 = Index Array(array=w262) -> (element=w260:string)  [unwired: 1 in]
                }
              }
            }
          }
          n104 = Greater Than 0?(x=w239) -> (x > 0?=w236:bool)
          n105 = Select(t="parent " ("pattern"), s=w236, f=w235) -> (s? t:f=w237:string)
          n106 = Select(t=w234, s=w236, f=w235) -> ()  [unwired: 1 out]
          n107 = Empty String/Path?(string/path=w241) -> (empty?=w240:bool)
        }
        n108 = case shown="\"utils\"" w231 {
          tunnel: [_ "private" ("Type") "protected" ("Type") "utils" ("Type")] -> w218
          frame Default {
          }
          frame "private" {
          }
          frame "protected" {
          }
          frame "utils" {
          }
        }
        n109 = property class="VI"(reference=w228, error in=w220) -> (reference out=w224:refnum<vi>, error out=w221:errorcluster, "VIType"=w227:T18)
        n110 = case shown="\"Control VI\"" w227 {
          tunnel: ["Control" ("pattern") "VI" ("pattern")] -> w226
          frame "Control VI" {
          }
          frame "Standard VI", Default {
          }
        }
        n111 = case shown="\"\"" w230 {
          selector: w230 -> [w267 _]
          tunnel: [w286 w401] -> w233
          tunnel: w229 -> [w285 w401]
          tunnel: w226 -> [w269 _]
          tunnel: w225 -> [w268 _]
          tunnel: w224 -> [w280 _]
          tunnel: w215 -> [w279 _]
          tunnel: w223 -> [w278 _]
          tunnel: w222 -> [w277 _]
          tunnel: w221 -> [w275 w400]
          tunnel: [w274 w400] -> w219
          tunnel: w218 -> [w273 _]
          tunnel: w214 -> [w272 _]
          tunnel: w211 -> [w266 _]
          frame Default {
            n112 = Build Path(base path=w279, name or relative path=w267) -> (appended path=w276:path)
            n113 = Format Into String(format string="This %s doesn't belong to a %s but there is a %s in this %s's %sfolder.\nDo you want to add this %s to the %s: %s?", w269, w268, w268, w269, w272, w269, w268, w267) -> (resulting string=w283:string)  [unwired: 2 in, 1 out]
            n114 = Format Into String(format string="Add %s to %s" ("T button name (\"OK\")"), w269, w268) -> (resulting string=w270:string)  [unwired: 2 in, 1 out]
            n115 = case shown="False" w266 {
              tunnel: w283 -> [w290 _]
              tunnel: "Ignore" ("F button name (\"Cancel\")") -> [w289 _]
              tunnel: [w288 _] -> w281
              tunnel: w270 -> [w287 _]
              frame False {
                n116 = Two Button Dialog(message=w290, 1:w289, 2:w287) -> (T button?=w288:bool)
              }
              frame True {
              }
            }
            n117 = case shown="True" w281 {
              tunnel: [w291 w303] -> w286
              tunnel: w285 -> [w291 w302]
              tunnel: w280 -> [_ _]
              tunnel: w278 -> [_ w301]
              tunnel: w277 -> [_ w300]
              tunnel: w276 -> [_ w299]
              tunnel: w275 -> [w292 w298]
              tunnel: [w292 w297] -> w274
              tunnel: w268 -> [_ w296]
              tunnel: [_ w294] -> _
              tunnel: w273 -> [_ w293]
              frame False {
              }
              frame True {
                n118 = case shown="\"class\", Default" w296 {
                  tunnel: w301 -> [w313 w347 w378]
                  tunnel: w300 -> [w306 w341 w373]
                  tunnel: w299 -> [w312 w346 w377]
                  tunnel: [w307 w342 w374] -> w295
                  tunnel: w298 -> [w311 w345 w376]
                  tunnel: [w310 w339 w371] -> w297
                  tunnel: w293 -> [w309 w344 w375]
                  frame "class", Default {
                    n119 = invoke class="App" method="LVClass.Open"(reference=w313, error in=w311, "Path"=w312) -> (error out=w308:errorcluster, "LVClass.Open"=w307:refnum<vi>)  [unwired: 1 in, 2 out]
                    n120 = case shown="Default" w309 {
                      selector: w309 -> [w324 _]
                      tunnel: w308 -> [w326 w336]
                      tunnel: w307 -> [w325 w337]
                      tunnel: w306 -> [w323 w333]
                      tunnel: [w322 w334] -> w305
                      tunnel: [w320 w335] -> w304
                      frame Default {
                        w328 = TRUE ("ExcludeDependencies")
                        n121 = invoke class="LVClassLibrary" method="Get All Descendents"(reference=w325, error in=w326, "Type"="Folder", "Exclude Dependencies"=w328, "ExcludeBuilds"=w328) -> (reference out=w316:refnum<vi>, error out=w321:errorcluster, "All Descendents"=w319:refnum<vi>[])  [unwired: 2 in, 4 out]
                        n122 = for {
                          tunnel: w319 -> [w332] mode=indexing
                          tunnel: [w330] -> w329 mode=indexing
                          n123 = property class="ProjectItem"(reference=w332) -> ("Name"=w331:string)  [unwired: 1 in, 2 out]
                          n124 = To Lower Case(string=w331) -> (all lower case string=w330:string)
                        }
                        n125 = Search 1D Array(1D array=w329, element=w324) -> (index of element=w318:i32)  [unwired: 1 in]
                        n126 = Less Than 0?(x=w318) -> (x < 0?=w317:bool)
                        n127 = Index Array(array=w319, index=w318) -> (element=w315:refnum<vi>)
                        n128 = Select(t=w316, s=w317, f=w315) -> (s? t:f=w314:refnum<vi>)
                        n129 = invoke class="ProjectItem" method="AddFile"(reference=w314, error in=w321, "Path"=w323) -> (error out=w320:errorcluster, "AddFile"=w322:refnum<vi>)  [unwired: 1 in, 2 out]
                        n130 = Close Reference(reference=w319, error in (no error)=w320) -> ()  [unwired: 1 out]
                      }
                      frame "" {
                        n131 = invoke class="LVClassLibrary" method="AddFile"(reference=w337, error in=w336, "Path"=w333) -> (error out=w335:errorcluster, "AddFile"=w334:refnum<vi>)  [unwired: 1 in, 2 out]
                      }
                    }
                    n132 = Close Reference(reference=w305, error in (no error)=w304) -> (error out=w310:errorcluster)
                  }
                  frame "library" {
                    n133 = invoke class="App" method="Library.Open"(reference=w347, error in=w345, "path"=w346) -> (error out=w343:errorcluster, "Open Library"=w342:refnum<vi>)  [unwired: 1 in, 2 out]
                    n134 = case shown="Default" w344 {
                      selector: w344 -> [w353 _]
                      tunnel: w343 -> [w355 w367]
                      tunnel: w342 -> [w354 w368]
                      tunnel: w341 -> [w352 w364]
                      tunnel: [w351 w365] -> w338
                      tunnel: [w349 w366] -> w340
                      frame Default {
                        w357 = TRUE ("ExcludeDependencies")
                        n135 = invoke class="Library" method="Get All Descendents"(reference=w354, error in=w355, "Type"="Folder", "Exclude Dependencies"=w357, "ExcludeBuilds"=w357) -> (error out=w350:errorcluster, "All Descendents"=w348:refnum<vi>[])  [unwired: 2 in, 5 out]
                        n136 = for {
                          tunnel: w348 -> [w363] mode=indexing
                          tunnel: [w361] -> w360 mode=indexing
                          n137 = property class="ProjectItem"(reference=w363) -> ("Name"=w362:string)  [unwired: 1 in, 2 out]
                          n138 = To Lower Case(string=w362) -> (all lower case string=w361:string)
                        }
                        n139 = Search 1D Array(1D array=w360, element=w353) -> (index of element=w358:i32)  [unwired: 1 in]
                        n140 = Index Array(array=w348, index=w358) -> (element=w359:refnum<vi>)
                        n141 = invoke class="ProjectItem" method="AddFile"(reference=w359, error in=w350, "Path"=w352) -> (error out=w349:errorcluster, "AddFile"=w351:refnum<vi>)  [unwired: 1 in, 2 out]
                        n142 = Close Reference(reference=w348, error in (no error)=w349) -> ()  [unwired: 1 out]
                      }
                      frame "" {
                        n143 = invoke class="Library" method="AddFile"(reference=w368, error in=w367, "Path"=w364) -> (error out=w366:errorcluster, "AddFile"=w365:refnum<vi>)  [unwired: 1 in, 2 out]
                      }
                    }
                    n144 = Close Reference(reference=w338, error in (no error)=w340) -> (error out=w339:errorcluster)
                  }
                  frame "X-control" {
                    n145 = invoke class="App" method="XControl.Open"(reference=w378, error in=w376, "Path"=w377) -> (error out=w369:errorcluster, "Open XControl"=w374:refnum<vi>)  [unwired: 1 in, 2 out]
                    n146 = case shown="Default" w375 {
                      selector: w375 -> [w384 _]
                      tunnel: w369 -> [w386 w398]
                      tunnel: w374 -> [w385 w399]
                      tunnel: w373 -> [w383 w395]
                      tunnel: [w382 w396] -> w370
                      tunnel: [w380 w397] -> w372
                      frame Default {
                        w388 = TRUE ("ExcludeDependencies")
                        n147 = invoke class="XCtlLib" method="Get All Descendents"(reference=w385, error in=w386, "Type"="Folder", "Exclude Dependencies"=w388, "ExcludeBuilds"=w388) -> (error out=w381:errorcluster, "All Descendents"=w379:refnum<vi>[])  [unwired: 2 in, 5 out]
                        n148 = for {
                          tunnel: w379 -> [w394] mode=indexing
                          tunnel: [w392] -> w391 mode=indexing
                          n149 = property class="ProjectItem"(reference=w394) -> ("Name"=w393:string)  [unwired: 1 in, 2 out]
                          n150 = To Lower Case(string=w393) -> (all lower case string=w392:string)
                        }
                        n151 = Search 1D Array(1D array=w391, element=w384) -> (index of element=w389:i32)  [unwired: 1 in]
                        n152 = Index Array(array=w379, index=w389) -> (element=w390:refnum<vi>)
                        n153 = invoke class="ProjectItem" method="AddFile"(reference=w390, error in=w381, "Path"=w383) -> (error out=w380:errorcluster, "AddFile"=w382:refnum<vi>)  [unwired: 1 in, 2 out]
                        n154 = Close Reference(reference=w379, error in (no error)=w380) -> ()  [unwired: 1 out]
                      }
                      frame "" {
                        n155 = invoke class="XCtlLib" method="AddFile"(reference=w399, error in=w398, "Path"=w395) -> (error out=w397:errorcluster, "AddFile"=w396:refnum<vi>)  [unwired: 1 in, 2 out]
                      }
                    }
                    n156 = Close Reference(reference=w370, error in (no error)=w372) -> (error out=w371:errorcluster)
                  }
                }
                n157 = Bundle By Name(cluster=w302, "LibraryRef"=w295) -> (w303:T6)
                n158 = invoke class="Library" method="Save"(reference=w295) -> (error out=w294:errorcluster)  [unwired: 3 in, 3 out]
              }
            }
          }
          frame "" {
          }
        }
      }
      frame "AnalyseFileName" {
        n159 = Unbundle By Name(w409) -> ("LibraryRef"=w407:refnum<vi>)
        n160 = Unbundle By Name(w409) -> ("Folder"=w415:path)
        n161 = local read "_VIPath"() -> (w411:path)
        n162 = Not A Number/Path/Refnum?(number/path/refnum=w415) -> (NaN/Path/Refnum?=w413:bool)
        n163 = Empty String/Path?(string/path=w415) -> (empty?=w414:bool)
        n164 = Not A Number/Path/Refnum?(number/path/refnum=w407) -> (NaN/Path/Refnum?=w408:bool)
        n165 = Or(x=w414, y=w413) -> (x .or. y?=w412:bool)
        n166 = case shown="False" w412 {
          tunnel: w409 -> [w438 w504]
          tunnel: [w437 w503] -> w417
          tunnel: [w436 w504] -> w416
          tunnel: w415 -> [w435 _]
          tunnel: w411 -> [w426 _]
          tunnel: w410 -> [w434 w503]
          tunnel: w408 -> [w433 _]
          tunnel: w407 -> [w432 _]
          tunnel: [w418 _] -> w405
          frame False {
            n167 = case shown="False" w433 {
              tunnel: [w469 w501] -> w437
              tunnel: w435 -> [w453 w497]
              tunnel: w426 -> [w454 w500]
              tunnel: [w459 w499] -> w429
              tunnel: [w467 w495] -> w430
              tunnel: [w466 w494] -> w431
              tunnel: w434 -> [w471 w498]
              tunnel: w432 -> [w472 _]
              tunnel: [w455 w496] -> w427
              tunnel: [w456 w493] -> w418
              frame False {
                n168 = property class="Library"(reference=w472, error in=w471) -> (error out=w469:errorcluster, "Name"=w465:string)  [unwired: 1 out]
                n169 = Strip Path(path=w454) -> (name=w468:string)  [unwired: 1 out]
                n170 = Match Pattern(string=w465, regular expression="\\2E[Ll][Vv][Ll][Ii][Bb]$") -> (before substring=w463:string)  [unwired: 1 in, 3 out]
                n171 = Match Pattern(string=w463, regular expression="\\2E[Ll][Vv][Cc][Ll][Aa][Ss][Ss]$") -> (before substring=w462:string, offset past match=w458:i32)  [unwired: 1 in, 2 out]
                n172 = Match Pattern(string=w462, regular expression="\\2E[Xx][Cc][Tt][Ll]$") -> (before substring=w461:string)  [unwired: 1 in, 3 out]
                n173 = call <resource>:"GDSIconEditor_FindPrefixInfo.vi"("_VIPath"=w454, "Folder"=w453) -> ("FolderFiles"=w448:path[], "Prefix"=w452:string, "Separator"=w451:string, "name"=w450:string, "FilePreFix+Separtor"=w449:string)  [unwired: 8 in, 1 out]
                n174 = Greater Or Equal To 0?(x=w458) -> (x >= 0?=w457:bool)
                n175 = case shown="True" w457 {
                  tunnel: w468 -> [_ w485]
                  tunnel: [w476 w481] -> w467
                  tunnel: [w475 w480] -> w466
                  tunnel: w461 -> [_ w479]
                  tunnel: [w477 w479] -> w459
                  tunnel: [w474 _] -> w456
                  tunnel: [w473 w478] -> w455
                  tunnel: w452 -> [w477 _]
                  tunnel: w451 -> [w476 _]
                  tunnel: w450 -> [w475 _]
                  tunnel: w449 -> [w474 _]
                  tunnel: w448 -> [w473 w478]
                  frame False {
                  }
                  frame True {
                    w481 = "[_\\s]+" ("Separator")
                    n176 = Concatenate Strings("^", w479, w481) -> (w492:string)
                    n177 = Match Pattern(string=w485, regular expression=w492) -> (before substring=w484:string, after substring=w483:string)  [unwired: 1 in, 2 out]
                    n178 = Concatenate Strings(w484, w483) -> (w482:string)
                    n179 = Match Pattern(string=w482, regular expression="\\2Evi$") -> (before substring=w488:string)  [unwired: 1 in, 3 out]
                    n180 = Match Pattern(string=w488, regular expression="\\2Ectl$") -> (before substring=w489:string)  [unwired: 1 in, 3 out]
                    n181 = Match Pattern(string=w489, regular expression="\\2Evit$") -> (before substring=w480:string)  [unwired: 1 in, 3 out]
                  }
                }
              }
              frame True {
                n182 = call <resource>:"GDSIconEditor_FindPrefixInfo.vi"("_VIPath"=w500, "Folder"=w497, "error in (no error)"=w498) -> ("FolderFiles"=w496:path[], "Prefix"=w499:string, "Separator"=w495:string, "name"=w494:string, "FilePreFix+Separtor"=w493:string, "error out"=w501:errorcluster)  [unwired: 7 in]
              }
            }
            n183 = for {
              tunnel: w427 -> [w440] mode=indexing
              shift-right: [w442] -> w425
              shift-left: path[] [] -> [w443]
              tunnel: w426 -> [w439]
              n184 = Not Equal?(x=w440, y=w439) -> (x != y?=w441:bool)
              n185 = case shown="True" w441 {
                tunnel: w443 -> [w444 w447]
                tunnel: [w444 w446] -> w442
                tunnel: w440 -> [_ w445]
                frame False {
                }
                frame True {
                  n186 = Build Array (concatenate)(w447, w445) -> (w446:path[])
                }
              }
            }
            n187 = Array Size(array=w425) -> (size(s)=w423:i32)
            n188 = Greater Than 0?(x=w423) -> (x > 0?=w422:bool)
            n189 = Select(t=u8 0, s=w422, f=u8 2 ("Disabled")) -> (s? t:f=w424:u8)
            n190 = property on="_ApplyHeaderToAll" class="Bool (strict)"("Disabled"=w424) -> ()  [unwired: 2 in, 2 out]
            n191 = call <resource>:"GDSIconEditor_SplitNameInRows.vi"("name"=w431) -> ("result string"=w419:string)
            n192 = Bundle By Name(cluster=w438, "VIs"=w425, "Prefix"=w429, "Separator"=w430, "StartMethodName"=w419) -> (w436:T6)
          }
          frame True {
            n193 = local write "_MethodIconName"("NoFilePath" ("Method Icon Name")) -> ()
          }
        }
        "_FilePrefixFound" <- w405
      }
      frame "Auto find header" {
        n194 = Unbundle By Name(w516) -> ("AppRef"=w514:refnum<vi>, "Scope"=w515:T3, "VIs"=w512:path[])
        n195 = Unbundle By Name(w516) -> ("LibraryRef"=w517:refnum<vi>)
        n196 = Unbundle By Name(w516) -> ("ViRef"=w513:refnum<vi>, "Scope"=w519:T3)
        n197 = To Variant(anything=w513) -> (Variant=w508:variant)
        n198 = for {
          tunnel: w512 -> [w523] mode=indexing
          tunnel: [w522] -> w511 mode=indexing
          n199 = To Variant(anything=w523) -> (Variant=w522:variant)
        }
        n200 = Build Array (concatenate)(w508, w511, w508) -> (w510:variant[])
        n201 = Not A Number/Path/Refnum?(number/path/refnum=w517) -> (NaN/Path/Refnum?=w518:bool)
        n202 = case shown="True" w518 {
          tunnel: [w528 w676] -> w507
          tunnel: [w527 w669] -> w521
          tunnel: w510 -> [_ w673]
          tunnel: w519 -> [_ _]
          tunnel: w520 -> [w526 w670]
          tunnel: w516 -> [w534 w677]
          tunnel: w517 -> [w525 _]
          tunnel: w515 -> [w530 _]
          tunnel: w514 -> [_ _]
          tunnel: w505 -> [w524 w656]
          frame False {
            n203 = disable-structure shown="Enabled" {
              disable-tunnel: [w538 w541] -> w532
              disable-tunnel: [w537 w540] -> w531
              disable-tunnel: w526 -> [w536 w541]
              disable-tunnel: w525 -> [w535 w540]
              frame Disabled {
                w539 = refnum<vi> refnum  # LVClassLibrary
                n204 = To More Specific Class(target class=w539, reference=w535, error in=w536) -> (specific class reference=w537:refnum<vi>, error out=w538:errorcluster)
              }
              frame Enabled {
              }
            }
            n205 = Bundle By Name(cluster=w534, "Header exists"=TRUE) -> (w529:T6)
            n206 = case shown="Error" w532 {
              selector: w532 -> [w582 _]
              tunnel: w531 -> [w581 _]
              tunnel: w530 -> [w590 _]
              tunnel: w529 -> [w580 w641]
              tunnel: [w579 w640] -> w528
              tunnel: [w576 w636] -> w527
              tunnel: w525 -> [_ w617]
              tunnel: w526 -> [_ w615]
              tunnel: w524 -> [w542 _]
              frame No Error {
                w588 = u8 32 ("x")
                w553 = u32 0
                n207 = call <resource>:"GDSLvClass_ReadClassColors.vi"("Library Refnum"=w581, "error in (no error)"=w582) -> ("Library Refnum"=w567:refnum<vi>, "LvClassIconSettings"=w560:T19, "LvClassIconSettingsFound"=w561:bool, "error out"=w575:errorcluster)  [unwired: 12 in, 2 out]
                n208 = Unbundle By Name(w560) -> ("ColorPrivate"=w556:u32, "ColorProtected"=w557:u32, "ColorPublic"=w558:u32, "Frame"=w555:u32, "Body Text"=w554:u32)
                n209 = case shown="\"Proteced\"" w590 {
                  tunnel: [w612 w613 w614] -> w574
                  tunnel: w558 -> [w612 _ _]
                  tunnel: w557 -> [_ w613 _]
                  tunnel: w556 -> [_ _ w614]
                  frame "Public", Default {
                  }
                  frame "Proteced" {
                  }
                  frame "Private" {
                  }
                }
                n210 = Unbundle By Name(w560) -> ("Frame thickness"=w559:u8, "ClassBodyIcon"=w544:string)
                n211 = call <resource>:"GDSLvIcon_AnalyseViIcon.vi"("ViRef/LvCLassRef/LvLibRef/ViPath/2D_Image"=w567, "error in (no error)"=w575) -> ("BodyTextColor"=w568:u32, "FrameColor"=w570:u32, "FrameThickness(1)"=w571:u32, "DefaultIcon"=w543:bool, "HeaderIcon"=w546:u8[][], "HeaderBkColor"=w545:u32, "BodyBkColor"=w569:u32, "error out"=w576:errorcluster)  [unwired: 5 in, 5 out]
                n212 = case shown="False" w561 {
                  tunnel: [w594 w611] -> w552
                  tunnel: w574 -> [_ w611]
                  tunnel: [w592 w610] -> w565
                  tunnel: w554 -> [_ w610]
                  tunnel: [w597 w609] -> w573
                  tunnel: w555 -> [_ w609]
                  tunnel: [w598 w608] -> w572
                  tunnel: w559 -> [_ w608]
                  tunnel: w571 -> [w598 _]
                  tunnel: w570 -> [w597 _]
                  tunnel: w569 -> [w595 _]
                  tunnel: w568 -> [w593 _]
                  tunnel: w543 -> [w596 _]
                  tunnel: w542 -> [w591 _]
                  frame False {
                    n213 = case shown="True" w596 {
                      tunnel: w595 -> [w600 _]
                      tunnel: [w600 w602] -> w594
                      tunnel: [w599 u32 0] -> w592
                      tunnel: w593 -> [w599 _]
                      tunnel: w591 -> [_ w601]
                      frame False {
                      }
                      frame True {
                        n214 = Array Size(array=w601) -> (size(s)=w603:i32)
                        n215 = Random Number (0-1)() -> (number: 0 to 1=w605:dbl)
                        n216 = Multiply(x=w603, y=w605) -> (x*y=w606:dbl)
                        n217 = Round Toward -Infinity(1:w606) -> (0:w604:dbl)
                        n218 = Index Array(array=w601, index=w604) -> (element=w602:u32)
                      }
                    }
                  }
                  frame True {
                  }
                }
                n219 = Multiply(x=w559, y=u8 2) -> (x*y=w586:u8)
                n220 = Array Size(array=w546) -> (size(s)=w583:i32[])
                n221 = local read "_BackgroundColor"() -> (w550:T2)
                n222 = Index Array(array=w583) -> (element #1=w585:i32)  [unwired: 2 in, 1 out]
                n223 = Equal?(x=w552, y=w565) -> (x = y?=w566:bool)
                n224 = Bundle(cluster=w550, "Color"=w552) -> (w551:T2)  [unwired: 1 in]
                n225 = Add(x=w585, y=w586) -> (x+y=w587:i32)
                n226 = Equal?(x=w552, y=w553) -> (x = y?=w564:bool)
                n227 = Increment(x=w587) -> (x+1=w589:i32)
                n228 = local write "_BackgroundColor"(w551) -> ()
                n229 = local read "_BodyTextColor"() -> (w547:T2)
                n230 = Select(t=u32 16777215, s=w564, f=w553) -> (s? t:f=w562:u32)
                n231 = Subtract(x=w588, y=w589) -> (x-y=w578:i32)
                n232 = Subtract(x=w588, y=w586) -> (x-y=w577:u8)
                n233 = Bundle By Name(cluster=w580, "FrameColor"=w573, "Frame thickness"=w572, "HeaderIcon"=w546, "HeaderBkColor"=w545, "BodyIconHeight"=w578, "BodyIconWidth"=w577, "ClassBodyIcon"=w544) -> (w579:T6)
                n234 = Select(t=w562, s=w566, f=w565) -> (s? t:f=w549:u32)
                n235 = Bundle(cluster=w547, "Color"=w549) -> (w548:T2)  [unwired: 1 in]
                n236 = local write "_BodyTextColor"(w548) -> ()
              }
              frame Error {
                w621 = refnum<vi> refnum  # Library
                w647 = u8 32 ("x")
                w629 = u32 0
                n237 = To More Specific Class(target class=w621, reference=w617, error in=w615) -> (specific class reference=w618:refnum<vi>, error out=w620:errorcluster)
                n238 = case shown="No Error" w620 {
                  selector: w620 -> [w649 _]
                  tunnel: [w650 w653] -> w619
                  tunnel: w618 -> [w650 _]
                  tunnel: w617 -> [_ w654]
                  tunnel: [w649 w652] -> w616
                  tunnel: w615 -> [_ w651]
                  frame No Error {
                  }
                  frame Error {
                    w655 = refnum<vi> refnum  # XControlLibrary
                    n239 = To More Specific Class(target class=w655, reference=w654, error in=w651) -> (specific class reference=w653:refnum<vi>, error out=w652:errorcluster)
                  }
                }
                n240 = call <resource>:"GDSLvIcon_AnalyseViIcon.vi"("ViRef/LvCLassRef/LvLibRef/ViPath/2D_Image"=w619, "error in (no error)"=w616) -> ("BodyTextColor"=w622:u32, "FrameColor"=w635:u32, "FrameThickness(1)"=w634:u32, "HeaderIcon"=w639:u8[][], "BodyBkColor"=w623:u32, "error out"=w636:errorcluster)  [unwired: 5 in, 7 out]
                n241 = Array Size(array=w639) -> (size(s)=w642:i32[])
                n242 = local read "_BackgroundColor"() -> (w627:T2)
                n243 = Multiply(x=w634, y=u8 2) -> (x*y=w645:u32)
                n244 = Equal?(x=w623, y=w622) -> (x = y?=w633:bool)
                n245 = Index Array(array=w642) -> (element #1=w644:i32)  [unwired: 2 in, 1 out]
                n246 = Bundle(cluster=w627, "Color"=w623) -> (w628:T2)  [unwired: 1 in]
                n247 = Add(x=w644, y=w645) -> (x+y=w646:u32)
                n248 = local write "_BackgroundColor"(w628) -> ()
                n249 = Equal?(x=w623, y=w629) -> (x = y?=w632:bool)
                n250 = Increment(x=w646) -> (x+1=w648:u32)
                n251 = Select(t=u32 16777215, s=w632, f=w629) -> (s? t:f=w630:u32)
                n252 = local read "_BodyTextColor"() -> (w624:T2)
                n253 = Select(t=w630, s=w633, f=w622) -> (s? t:f=w626:u32)
                n254 = Subtract(x=w647, y=w648) -> (x-y=w638:u32)
                n255 = Subtract(x=w647, y=w645) -> (x-y=w637:u32)
                n256 = Bundle(cluster=w624, "Color"=w626) -> (w625:T2)  [unwired: 1 in]
                n257 = local write "_BodyTextColor"(w625) -> ()
                n258 = Bundle By Name(cluster=w641, "FrameColor"=w635, "Frame thickness"=w634, "HeaderIcon"=w639, "BodyIconHeight"=w638, "BodyIconWidth"=w637) -> (w640:T6)
              }
            }
          }
          frame True {
            w686 = u8 32 ("x")
            n259 = for {
              tunnel: [w718] -> w684
              tunnel: [w717] -> w663
              tunnel: w673 -> [w716] mode=indexing
              tunnel: [w715] -> w672
              tunnel: [w714] -> w671
              tunnel: [w713] -> w660
              tunnel: w670 -> [w712]
              tunnel: [w711] -> w669
              tunnel: [w710] -> w658
              tunnel: [w709] -> w659
              tunnel: [w708] -> w657
              stop <- w710 stop-if-true
              n260 = call <resource>:"GDSLvIcon_AnalyseViIcon.vi"("ViRef/LvCLassRef/LvLibRef/ViPath/2D_Image"=w716, "error in (no error)"=w712) -> ("BodyTextColor"=w713:u32, "FrameColor"=w714:u32, "FrameThickness(1)"=w715:u32, "ValidHeaderIcon"=w710:bool, "DefaultIcon"=w708:bool, "HeaderIcon"=w718:u8[][], "HeaderBkColor"=w709:u32, "BodyBkColor"=w717:u32, "error out"=w711:errorcluster)  [unwired: 5 in, 4 out]
            }
            n261 = case shown="False" w657 {
              tunnel: w663 -> [w692 _]
              tunnel: [w691 w703] -> w662
              tunnel: [w690 u32 0] -> w661
              tunnel: w660 -> [w688 _]
              tunnel: w656 -> [_ w701]
              frame False {
                n262 = Equal?(x=w692, y=w688) -> (x = y?=w693:bool)
                n263 = Equal?(x=w688, y=u32 0) -> (x = y?=w689:bool)
                n264 = case shown="True" w693 {
                  tunnel: w688 -> [w694 _]
                  tunnel: w692 -> [w695 w700]
                  tunnel: [w695 w700] -> w691
                  tunnel: [w694 w698] -> w690
                  tunnel: w689 -> [_ w699]
                  frame False {
                  }
                  frame True {
                    n265 = Select(t=u32 16777215, s=w699, f=u32 0) -> (s? t:f=w698:u32)
                  }
                }
              }
              frame True {
                n266 = Array Size(array=w701) -> (size(s)=w704:i32)
                n267 = Random Number (0-1)() -> (number: 0 to 1=w706:dbl)
                n268 = Multiply(x=w704, y=w706) -> (x*y=w707:dbl)
                n269 = Round Toward -Infinity(1:w707) -> (0:w705:dbl)
                n270 = Index Array(array=w701, index=w705) -> (element=w703:u32)
              }
            }
            n271 = Array Size(array=w684) -> (size(s)=w685:i32[])
            n272 = Index Array(array=w685) -> (element #1=w668:i32)  [unwired: 2 in, 1 out]
            n273 = Multiply(x=w672, y=u8 2) -> (x*y=w674:u32)
            n274 = local read "_BodyTextColor"() -> (w678:T2)
            n275 = Equal To 0?(x=w668) -> (x = 0?=w667:bool)
            n276 = local read "_BackgroundColor"() -> (w681:T2)
            n277 = Add(x=w668, y=w674) -> (x+y=w665:u32)
            n278 = Bundle(cluster=w681, "Color"=w662) -> (w680:T2)  [unwired: 1 in]
            n279 = Increment(x=w665) -> (x+1=w666:u32)
            n280 = local write "_BackgroundColor"(w680) -> ()
            n281 = Select(t=w665, s=w667, f=w666) -> (s? t:f=w664:u32)
            n282 = Bundle(cluster=w678, "Color"=w661) -> (w679:T2)  [unwired: 1 in]
            n283 = Subtract(x=w686, y=w664) -> (x-y=w683:u32)
            n284 = Subtract(x=w686, y=w674) -> (x-y=w682:u32)
            n285 = local write "_BodyTextColor"(w679) -> ()
            n286 = Bundle By Name(cluster=w677, "FrameColor"=w671, "Frame thickness"=w672, "HeaderIcon"=w684, "BodyIconHeight"=w683, "BodyIconWidth"=w682, "Header exists"=w658, "HeaderBkColor"=w659) -> (w676:T6)
          }
        }
        n287 = Unbundle By Name(w507) -> ("Header exists"=w506:bool)
        n288 = property on="_HideHeader" class="Bool (strict)"("Visible"=w506) -> ()  [unwired: 2 in, 2 out]
      }
      frame "UseBeforePicture" {
        (unwired) "UpdateIcon"
        w737 = u32 0
        w750 = u8 32 ("x")
        (unwired) "DoIconTextOCR"
        n289 = Unbundle By Name(w752) -> ("ViRef"=w729:refnum<vi>)
        n290 = call <resource>:"GDSLvIcon_AnalyseViIcon.vi"("ViRef/LvCLassRef/LvLibRef/ViPath/2D_Image"=w729, "error in (no error)"=w727) -> ("BodyTextColor"=w723:u32, "FrameColor"=w742:u32, "FrameThickness(1)"=w728:u32, "DefaultIcon"=w724:bool, "HeaderIcon"=w731:u8[][], "HeaderBkColor"=w730:u32, "BodyIcon"=w726:u8[][], "BodyBkColor"=w722:u32, "error out"=w753:errorcluster)  [unwired: 5 in, 4 out]
        n291 = case shown="True" w724 {
          tunnel: w722 -> [w756 _]
          tunnel: [w756 w758] -> w719
          tunnel: [w755 u32 0] -> w721
          tunnel: w723 -> [w755 _]
          tunnel: w720 -> [_ w757]
          frame False {
          }
          frame True {
            n292 = Array Size(array=w757) -> (size(s)=w759:i32)
            n293 = Random Number (0-1)() -> (number: 0 to 1=w761:dbl)
            n294 = Multiply(x=w759, y=w761) -> (x*y=w762:dbl)
            n295 = Round Toward -Infinity(1:w762) -> (0:w760:dbl)
            n296 = Index Array(array=w757, index=w760) -> (element=w758:u32)
          }
        }
        n297 = Array Size(array=w731) -> (size(s)=w745:i32[])
        n298 = local read "_BackgroundColor"() -> (w735:T2)
        n299 = Multiply(x=w728, y=u8 2) -> (x*y=w748:u32)
        n300 = Equal?(x=w719, y=w721) -> (x = y?=w741:bool)
        n301 = Bundle(cluster=w735, "Color"=w719) -> (w736:T2)  [unwired: 1 in]
        n302 = Index Array(array=w745) -> (element #1=w747:i32)  [unwired: 2 in, 1 out]
        n303 = local write "_BackgroundColor"(w736) -> ()
        n304 = Add(x=w747, y=w748) -> (x+y=w749:u32)
        n305 = Increment(x=w749) -> (x+1=w751:u32)
        n306 = Equal?(x=w719, y=w737) -> (x = y?=w740:bool)
        n307 = Select(t=u32 16777215, s=w740, f=w737) -> (s? t:f=w738:u32)
        n308 = Subtract(x=w750, y=w751) -> (x-y=w744:u32)
        n309 = Subtract(x=w750, y=w748) -> (x-y=w743:u32)
        n310 = Select(t=w738, s=w741, f=w721) -> (s? t:f=w734:u32)
        n311 = local read "_BodyTextColor"() -> (w732:T2)
        n312 = Bundle(cluster=w732, "Color"=w734) -> (w733:T2)  [unwired: 1 in]
        n313 = Bundle By Name(cluster=w752, "FrameColor"=w742, "Frame thickness"=w728, "HeaderIcon"=w731, "HeaderBkColor"=w730, "BodyIcon"=w726, "BodyIconHeight"=w744, "BodyIconWidth"=w743) -> (w754:T6)
        n314 = local write "_BodyTextColor"(w733) -> ()
      }
      frame "DoIconTextOCR", "DoIconTextOCR_Before" {
        # "First Time and OCR Text Found"
        n315 = Unbundle By Name(w774) -> ("FirstTime"=w767:bool, "StartMethodName"=w775:string, "ViRef"=w783:refnum<vi>)
        n316 = call <resource>:"GDSLvIcon_AnalyseViIcon.vi"("ViRef/LvCLassRef/LvLibRef/ViPath/2D_Image"=w783, "DoATextOCR(False)"=TRUE, "error in (no error)"=w785) -> ("BodyText(OCR)"=w770:string, "error out"=w786:errorcluster)  [unwired: 4 in, 11 out]
        n317 = call <resource>:"GOOP_OCREvaluation.vi"("OcrText"=w770, "Viname"=w775) -> ("Match"=w765:bool)  [unwired: 9 in]
        n318 = Not Equal?(x=w781, y="DoIconTextOCR_Before") -> (x != y?=w779:bool)
        n319 = Empty String/Path?(string/path=w770) -> (empty?=w769:bool)
        n320 = Compound Arithmetic op=AND(w767, invert w769) -> (w771:bool)
        n321 = local read "_OCR"() -> (w764:bool)
        n322 = And(x=w767, y=w765) -> (x .and. y?=w766:bool)
        n323 = Or(x=w766, y=w764) -> (x .or. y?=w768:bool)
        n324 = Select(t=w770, s=w768, f=w775) -> (s? t:f=w782:string)
        n325 = case shown="True" w771 {
          tunnel: w765 -> [_ w787]
          frame False {
          }
          frame True {
            w788 = FALSE ("Boolean Text.Font:Bold")
            n326 = property on="_OCR" class="Bool (strict)"("BoolText.FontBold"=w788, "BoolText.FontUnder"=w788, "Visible"=TRUE, "Value"=w787) -> ()  [unwired: 2 in, 2 out]
          }
        }
        n327 = local write "_MethodIconName"(w782) -> ()
        n328 = Bundle By Name(cluster=w774, "FirstTime"=FALSE) -> (w773:T6)
        n329 = Select(t="GuessIconSize", s=w779, f="UpdateIcon,ShowLayoutChange") -> (s? t:f=w776:string)
      }
      frame "GuessIconSize" {
        n330 = Unbundle By Name(w798) -> ("ViRef"=w792:refnum<vi>)
        n331 = property class="VI"(reference=w792) -> ("VIType"=w791:T18)  [unwired: 1 in, 2 out]
        n332 = case shown="Default" w791 {
          tunnel: w800 -> [w805 w820]
          tunnel: [w805 w819] -> w799
          tunnel: [0 ("StartRow") w817] -> w796
          tunnel: [w806 w816] -> w795
          tunnel: [i32[] [] ("ConnectorPaneHeight") w815] -> w794
          tunnel: [TRUE FALSE] -> w793
          tunnel: w792 -> [_ w809]
          tunnel: [_ TRUE] -> w790
          frame "Control VI", "Polymorphic VI" {
            w806 = u16 0 items=["Full", "1 c-term high", "2 c-term high", "3 c-term high"] ("_IconSize")
          }
          frame Default {
            n333 = call <resource>:"GOOP_GetControlRearrangement.vi"("VI Refnum"=w809, "_IconSize"=IconSize."Full" ("NewIconSize"), "error in (no error)"=w820) -> ("StartRow"=w817:i32, "ControlsToMove"=w811:T20, "ConnectorPaneHeight"=w815:i32[], "NumberOfTerminalAtStart"=w813:i32, "error out"=w819:errorcluster)  [unwired: 10 in, 2 out]
            n334 = Array Size(array=w811) -> (size(s)=w810:i32)
            n335 = Equal To 0?(x=w810) -> ()  [unwired: 1 out]
            n336 = Array Size(array=w815) -> (size(s)=w814:i32)
            n337 = Equal?(x=w814, y=w813) -> (x = y?=w812:bool)
            n338 = case shown="True" w812 {
              tunnel: [w822 w827] -> w816
              tunnel: w813 -> [w821 _]
              frame False {
                n339 = case shown="3" w821 {
                  tunnel: [w823 w824 w825 w826] -> w822
                  frame 1 {
                    w823 = u16 1 items=["Full", "1 c-term high", "2 c-term high", "3 c-term high"] ("_IconSize")
                  }
                  frame 2 {
                    w824 = u16 2 items=["Full", "1 c-term high", "2 c-term high", "3 c-term high"] ("_IconSize")
                  }
                  frame 3 {
                    w825 = u16 3 items=["Full", "1 c-term high", "2 c-term high", "3 c-term high"] ("_IconSize")
                  }
                  frame Default {
                    w826 = u16 0 items=["Full", "1 c-term high", "2 c-term high", "3 c-term high"] ("_IconSize")
                  }
                }
              }
              frame True {
                w827 = u16 0 items=["Full", "1 c-term high", "2 c-term high", "3 c-term high"] ("_IconSize")
              }
            }
          }
        }
        n340 = property on="_IconSize" class="Ring (strict)"("Visible"=w790) -> ()  [unwired: 2 in, 2 out]
        n341 = local write "_IconSize"(w795) -> ()
        n342 = Bundle By Name(cluster=w798, "StartRow"=w796, "NoControlsToMove"=w793, "ConnectorPaneHeight"=w794, "StartIconSize"=w795) -> (w797:T6)
      }
      frame "Generate icon" {
        n343 = Unbundle By Name(w831) -> ("Scope"=w832:T3)  [unwired: 1 out]
        n344 = case shown="True" TRUE {
          tunnel: w834 -> [w835 w890]
          tunnel: [w835 w889] -> w833
          tunnel: w832 -> [_ _]
          tunnel: w831 -> [w836 w858]
          tunnel: [w836 w886] -> w830
          frame False {
          }
          frame True {
            n345 = Unbundle By Name(w858) -> ("Frame thickness"=w848:i32, "ConnectorPaneHeight"=w874:i32[], "BodyIconHeight"=w873:i32, "BodyIconWidth"=w869:i32)
            n346 = Unbundle By Name(w858) -> ("StartIconSize"=w866:u16, "StartRow"=w862:i32, "FrameColor"=w867:u32, "Frame thickness"=w879:i32, "HeaderIcon"=w872:u8[][])
            n347 = local read "_MethodIconName"() -> (w887:string)
            n348 = local read "_FontCapitalOnly"() -> (w888:bool)
            n349 = local read "_FontCompression"() -> (w875:enum16{"Auto", "On", "Off"})
            n350 = local read "_IconSize"() -> (w865:u16)
            n351 = local read "_HideHeader"() -> (w837:bool)
            n352 = Not Equal?(x=w866, y=w865) -> (x != y?=w864:bool)
            n353 = call <resource>:"GDSIconEditor_IconSizeAdjustment.vi"("BodyIconHeightIn"=w873, "HideHeader"=w837, "ConnectorPaneHeight"=w874, "Frame thickness"=w848, "_IconSize"=w865, "HeaderIconIn"=w872) -> ("HeaderIconOut"=w871:u8[][], "BodyIconHeightOut"=w868:u32, "ImageRows"=w870:i32)  [unwired: 3 in]
            n354 = Select(t=0, s=w864, f=w862) -> (s? t:f=w861:i32)
            n355 = local read "_TextAlignment"() -> (w859:u16)
            n356 = Unbundle By Name(w858) -> ("OldOffset.X"=w855:i32, "OldOffset.Y"=w850:i32, "CurrentIcon"=w844:T21)
            n357 = local read "_BackgroundColor"() -> (w885:T2)
            n358 = Unbundle By Name(w858) -> ("Offset"=w854:cluster{"X":i32, "Y":i32})
            n359 = local read "_BodyTextColor"() -> (w883:T2)
            n360 = Bundle By Name(cluster=T10 {"Text"="", "Allow Only Capital Chars"=FALSE, "Compression"=enum."Auto", "Alignment"=enum."Center"} ("IconTextDataType"), "Text"=w887, "Allow Only Capital Chars"=w888, "Compression"=w875, "Alignment"=w859) -> (w881:T10)
            n361 = Unbundle By Name(w854) -> ("X"=w853:i32, "Y"=w849:i32)
            n362 = Unbundle By Name(w883) -> ("Color"=w847:u32)
            n363 = Unbundle By Name(w885) -> ("Color"=w884:u32)
            n364 = call <resource>:"GDSLvIcon_GenerateIconText.vi"("Text"=w881, "TextPixelHeight(5-30)"=w868, "Foreground color"=w847, "Background color"=w884, "error in (no error)"=w890, "Offset"=w854, "Text Pixel width(32-FrameThicknes*2))"=w869) -> ("X-Limited"=w857:bool, "Y-Limited"=w852:bool, "TextOut"=w845:u8[][], "TextBounds"=w843:T22, "error out"=w880:errorcluster)  [unwired: 8 in]
            n365 = Select(t=w855, s=w857, f=w853) -> (s? t:f=w856:i32)
            n366 = Select(t=w850, s=w852, f=w849) -> (s? t:f=w851:i32)
            n367 = call <resource>:"GDSLvIcon_CreateIconPicture.vi"("FrameColor"=w867, "FrameThickness(1)"=w879, "HeaderIconIn"=w871, "BodyIconIn"=w845, "error in (no error)"=w880, "ImageRows(32)"=w870, "BigSizeIcon(x6)"=4, "RowStart(0)"=w861, "BgIcon"=w844) -> ("WholeIconOut"=w877:u8[][], "IconPictureOut"=→"_After":picture, "LargeIconPictureOut(x6)"=→"_IconPreview":picture, "BodyOffset"=w841:cluster{"X":i32, "Y":i32}, "error out"=w889:errorcluster)  [unwired: 5 in, 1 out]
            n368 = Unbundle(w841) -> ("X"=w838:i32, "Y"=w839:i32)
            n369 = Bundle("Y"=w839, "X"=w838, "Y"=w839, "X"=w838) -> (w840:cluster{"Y":i32, "X":i32, "Y":i32, "X":i32})  [unwired: 1 in]
            n370 = Add(x=w840, y=w843) -> (x+y=w842:cluster{i32, i32, i32, i32})
            n371 = Bundle By Name(cluster=w858, "Offset.X"=w856, "Offset.Y"=w851, "Icon exist"=TRUE, "IconOut"=w877, "BodyIcon"=w845, "TextBounds"=w842) -> (w886:T6)
          }
        }
      }
      frame "UpdateIcon", "UpdateIcon,ShowLayoutChange" {
        w917 = T21 {"BgIcon"=[], "BgIconOffset"={"X"=0, "Y"=0}, "BgIconMask"=[], "ColorsOkayforiconToBeOnTopOf"=[]}  # BgIcon
        n372 = Unbundle By Name(w907) -> ("Frame thickness"=w922:i32, "ConnectorPaneHeight"=w935:i32[], "BodyIconHeight"=w934:i32, "BodyIcon"=w918:u8[][])
        n373 = Unbundle By Name(w907) -> ("StartIconSize"=w928:u16, "StartRow"=w924:i32, "FrameColor"=w929:u32, "Frame thickness"=w937:i32, "HeaderIcon"=w931:u8[][])
        n374 = local read "_BackgroundColor"() -> (w914:T2)
        n375 = local read "_IconSize"() -> (w927:u16)
        n376 = Unbundle By Name(w914) -> ("Color"=w909:u32)
        n377 = Unbundle By Name(w907) -> ("BgIcon"=w916:u8[][], "BgIconOffset"=w915:cluster{"X":i32, "Y":i32}, "BgIconMask"=w912:u8[], "HeaderBkColor"=w911:u32)
        n378 = case shown="Default" w927 {
          tunnel: w931 -> [w961 _]
          tunnel: [w961 _] -> w892
          frame Default {
          }
          frame 1 {
          }
        }
        n379 = Not Equal?(x=w928, y=w927) -> (x != y?=w926:bool)
        n380 = Array Size(array=w892) -> (size(s)=w933:i32[])
        n381 = Index Array(array=w933) -> (element=w932:i32)  [unwired: 1 in]
        n382 = call <resource>:"GDSLvIcon_Convert24bitTo8bitColor.vi"("Color 24bit In"=w911) -> ("Color out(256)"=w910:u8)  [unwired: 15 in, 3 out]
        n383 = call <resource>:"GDSLvIcon_Convert24bitTo8bitColor.vi"("Color 24bit In"=w909) -> ("Color out(256)"=w908:u8)  [unwired: 15 in, 3 out]
        n384 = Select(t=0, s=w926, f=w924) -> (s? t:f=w923:i32)
        n385 = local read "_HideHeader"() -> (w894:bool)
        n386 = Multiply(x=w922, y=u32 2) -> (x*y=w921:u32)
        n387 = case shown="1" w927 {
          selector: w927 -> [_ w951 _]
          tunnel: w934 -> [_ _ _]
          tunnel: w935 -> [_ w956 w959]
          tunnel: [32 ("ImageRows(32)") w950 w960] -> w930
          tunnel: w932 -> [_ w954 _]
          tunnel: w921 -> [_ w953 w957]
          frame 0 {
          }
          frame Default {
            n388 = Decrement(x=w951) -> ()  [unwired: 1 out]
            n389 = Array Subset(array=w956, length=w951) -> (w955:i32[])  [unwired: 1 in]
            n390 = Add Array Elements(numeric array=w955) -> (sum=w950:i32)
            n391 = Increment(x=w953) -> (x+1=w952:u32)
            n392 = Compound Arithmetic op=ADD(w952, w954, w950) -> ()  [unwired: 1 out]
          }
          frame 1 {
            n393 = Index Array(array=w959) -> (element=w958:i32)  [unwired: 1 in]
            n394 = Compound Arithmetic op=ADD(w957, w958) -> (w960:u32)
          }
        }
        n395 = stacked-sequence {
          tunnel: w902 -> [w943]
          tunnel: [w943] -> w901
          tunnel: [w942] -> w897
          frame #0 {
            n396 = Tick Count (ms)() -> (millisecond timer value=w942:u32)
          }
        }
        n397 = Build Array(w910, w908) -> (w913:u8[])
        n398 = Bundle By Name(cluster=w917, "BgIcon"=w916, "BgIconOffset"=w915, "BgIconMask"=w912, "ColorsOkayforiconToBeOnTopOf"=w913) -> (w905:T21)
        n399 = Select(t=u8[][] [], s=w894, f=w892) -> (s? t:f=w893:u8[][])
        n400 = call <resource>:"GDSLvIcon_CreateIconPicture.vi"("FrameColor"=w929, "FrameThickness(1)"=w937, "HeaderIconIn"=w893, "BodyIconIn"=w918, "error in (no error)"=w901, "ImageRows(32)"=w930, "BigSizeIcon(x6)"=4, "RowStart(0)"=w923, "BgIcon"=w905) -> ("WholeIconOut"=w904:u8[][], "IconPictureOut"=w920:picture, "LargeIconPictureOut(x6)"=w919:picture, "error out"=w900:errorcluster)  [unwired: 5 in, 2 out]
        n401 = Bundle By Name(cluster=w907, "CurrentIcon"=w905, "IconOut"=w904) -> (w906:T6)
        n402 = local write "_IconPreview"(w919) -> ()
        n403 = local write "_After"(w920) -> ()
        n404 = case shown="Default" w903 {
          tunnel: ["ShowLayoutChange" ("item tag") w946] -> w939
          tunnel: w895 -> [_ w945]
          frame "UpdateIcon,ShowLayoutChange" {
          }
          frame Default {
            n405 = case shown="True" w945 {
              tunnel: ["Idle" ("item tag") "Apply icon"] -> w946
              frame False {
              }
              frame True {
              }
            }
          }
        }
        n406 = stacked-sequence {
          tunnel: w900 -> [w941]
          tunnel: [w941] -> w899
          tunnel: [w940] -> w898
          frame #0 {
            n407 = Tick Count (ms)() -> (millisecond timer value=w940:u32)
          }
        }
        n408 = Subtract(x=w898, y=w897) -> (x-y=w896:u32)
      }
      frame "ShowLayoutChange" {
        (unwired) u16 1 items=["Full", "1 c-term high", "2 c-term high", "3 c-term high"] ("_IconSize")
        n409 = Unbundle By Name(w967) -> ("TermWindowOpen"=w965:bool, "NoControlsToMove"=w969:bool, "StartIconSize"=w972:u16)
        n410 = Unbundle By Name(w967) -> ("ViRef"=w978:refnum<vi>)
        n411 = local read "_IconSize"() -> (w976:u16)
        n412 = Equal To 0?(x=w972) -> (x = 0?=w973:bool)
        n413 = Equal To 0?(x=w976) -> (x = 0?=w977:bool)
        n414 = Select(t=u16 6, s=w973, f=w972) -> (s? t:f=w970:u16)
        n415 = Select(t=u16 6, s=w977, f=w976) -> (s? t:f=w971:u16)
        n416 = Less?(x=w971, y=w970) -> (x < y?=w968:bool)
        n417 = Compound Arithmetic op=AND(invert w969, w968) -> (w964:bool)
        n418 = case shown="True" w964 {
          tunnel: w981 -> [w985 w993]
          tunnel: [w984 w991] -> w980
          tunnel: w979 -> [w987 w992]
          tunnel: w978 -> [_ w990]
          tunnel: w976 -> [_ w989]
          tunnel: w965 -> [_ w988]
          frame False {
            n419 = Enqueue Element(queue=w987, element=cluster{"Message":string, "Picture":picture} {"Message"="Hide", "Picture"=bytes[0]}, error in (no error)=w985) -> (error out=w984:errorcluster)  [unwired: 1 in, 2 out]
          }
          frame True {
            n420 = case shown="False" w988 {
              tunnel: w993 -> [w1005 w1006]
              tunnel: w992 -> [w1004 _]
              tunnel: [w1000 w1006] -> w991
              tunnel: w990 -> [w999 _]
              tunnel: w989 -> [w998 _]
              frame False {
                n421 = local read "_Icons"() -> (w997:bool)
                n422 = call <resource>:"GOOP_GetControlRearrangement.vi"("VI Refnum"=w999, "_IconSize"=w998, "error in (no error)"=w1005) -> ("LayoutPicture"=w1003:picture, "error out"=w1001:errorcluster)  [unwired: 10 in, 5 out]
                n423 = Select(t=cluster{"Message":string, "Picture":picture} {"Message"="ShowLeftSide", "Picture"=bytes[0]} ("element"), s=w997, f=cluster{"Message":string, "Picture":picture} {"Message"="ShowRightSide", "Picture"=bytes[0]} ("element")) -> (s? t:f=w994:cluster{"Message":string, "Picture":picture})
                n424 = Bundle By Name(cluster=w994, "Picture"=w1003) -> (w1002:cluster{"Message":string, "Picture":picture})
                n425 = Enqueue Element(queue=w1004, element=w1002, error in (no error)=w1001) -> (error out=w1000:errorcluster)  [unwired: 1 in, 2 out]
              }
              frame True {
              }
            }
          }
        }
        n426 = Bundle By Name(cluster=w967, "LayoutChangeExist"=w964, "TermWindowOpen"=w964) -> (w966:T6)
        n427 = case shown="True" w962 {
          tunnel: ["Idle" ("item tag") "Apply icon"] -> w963
          frame False {
          }
          frame True {
          }
        }
      }
      frame "", "Idle" {
        n428 = local read "_VIPath"() -> (w1024:path)
        n429 = Unbundle By Name(w1022) -> ("IconSelected"=w1008:i32, "IconDropped"=w1009:i32, "Icon exist"=w1023:bool)
        n430 = Not A Number/Path/Refnum?(number/path/refnum=w1024) -> (NaN/Path/Refnum?=w1034:bool)
        n431 = Empty String/Path?(string/path=w1024) -> (empty?=w1033:bool)
        n432 = local read "_ApplyHeaderToAll"() -> (w1020:bool)
        n433 = Compound Arithmetic op=AND(invert w1034, invert w1033) -> (w1013:bool)
        n434 = Not(x=w1013) -> (.not. x?=w1012:bool)
        n435 = Not(x=w1013) -> (.not. x?=w1030:bool)
        n436 = And(x=w1023, y=w1013) -> (x .and. y?=w1025:bool)
        n437 = Select(t=u8 0 ("Disabled"), s=w1030, f=u8 2) -> (s? t:f=w1027:u8)
        n438 = Select(t=u8 2 ("Disabled"), s=w1012, f=u8 0) -> (s? t:f=w1016:u8)
        n439 = property on="_ViNotSavedMessage" class="Str"("Visible"=w1012) -> ()  [unwired: 2 in, 2 out]
        n440 = property class="VI"("Front Panel.Open"=TRUE ("Front Panel Window:Open")) -> ()  [unwired: 2 in, 2 out]
        n441 = property on="_VIPath" class="Path"("Disabled"=w1027) -> ()  [unwired: 2 in, 2 out]
        n442 = Select(t=1000, s=w1020, f=-1) -> (s? t:f=w1019:i32)
        n443 = Select(t=u8 0 ("Disabled"), s=w1025, f=u8 2) -> (s? t:f=w1026:u8)
        n444 = property on="_ApplyHeaderToAll" class="Bool (strict)"("Disabled"=w1016) -> ()  [unwired: 2 in, 2 out]
        n445 = property on="Accept" class="Bool"("Disabled"=w1026) -> ()  [unwired: 2 in, 2 out]
        n446 = event shown="[6] \"Icons\", \"DragIcon\": Mouse Move" {
          selector: _ -> [_ _ _ _ _ _ _ _ _ _ _ _ _ _ _ _ _ _ _ _ _ _ _ _ _ _ _ _ _ _ _ _ _ _]
          dyn-events: _ -> [_ _ _ _ _ _ _ _ _ _ _ _ _ _ _ _ _ _ _ _ _ _ _ _ _ _ _ _ _ _ _ _ _ _]
          timeout: w1019 -> [_ _ _ _ _ _ _ _ _ _ _ _ _ _ _ _ _ _ _ _ _ _ _ _ _ _ _ _ _ _ _ _ _ _]
          tunnel: ["Generate icon" "UseBeforePicture" ("t") w1052 w1117 "ReadIcons" w1142 w1147 "DrawIcons:NoBusy" ("y") w1186 _ _ _ "GetImageData" ("y") "UpdateIcon" ("y") w1285 "Idle" ("t") "Idle" ("t") _ "Generate icon" _ _ "DoIconTextOCR" ("t") "Generate icon" "Generate icon" "Idle" "AnalyseFileName" "UpdateApplyToAllText" "Template VI" "Idle" w1399 "Apply icon" w1415 "Exit" "Exit"] -> w1035
          tunnel: w1022 -> [_ w1040 w1058 w1104 _ _ w1145 _ w1184 _ w1231 w1237 _ w1266 w1268 _ w1330 _ _ _ _ _ _ _ _ w1380 _ _ _ w1397 _ w1411 _ _]
          tunnel: w1022 -> [w1037 w1042 w1057 w1120 w1137 w1139 w1149 w1182 w1190 w1229 w1234 w1239 w1259 w1263 w1287 w1327 w1328 w1333 w1336 w1338 w1340 w1343 w1345 w1356 w1359 w1375 w1381 w1383 w1385 w1398 w1408 w1414 w1420 w1422]
          tunnel: [w1037 w1042 w1056 w1120 w1137 w1139 w1148 w1182 w1189 w1228 w1233 w1238 w1258 w1262 w1286 w1326 w1328 w1333 w1335 w1338 w1340 w1343 w1345 w1355 w1359 w1370 w1381 w1383 w1385 w1398 w1408 w1413 w1420 w1422] -> w1021
          tunnel: w1011 -> [_ _ _ w1114 _ _ _ _ _ _ _ _ _ _ _ _ _ _ _ _ _ _ _ _ _ _ _ _ _ _ _ _ _ _]
          tunnel: w1010 -> [_ _ _ w1119 _ _ _ _ _ _ _ _ _ _ _ _ _ _ _ _ _ _ _ _ _ _ _ _ _ _ _ _ _ _]
          tunnel: w1009 -> [_ _ _ _ _ _ _ _ _ _ _ _ _ _ _ _ _ _ _ _ _ _ _ _ _ _ _ _ _ _ _ _ _ _]
          tunnel: w1008 -> [_ _ _ _ _ _ _ _ _ _ _ _ _ _ _ _ _ _ _ _ _ _ _ _ _ _ _ _ _ _ _ _ _ _]
          event "_MethodIconName": Value Change {
            n447 = event-data() -> ()  [unwired: 1 in, 6 out]
          }
          event "_Before": Mouse Down {
            n448 = event-data() -> ()  [unwired: 1 in, 8 out]
            n449 = Unbundle By Name(w1040) -> ("StartIconSize"=w1039:u16)
            n450 = local write "_IconSize"(w1039) -> ()
          }
          event Key Down? {
            (unwired) TRUE
            n451 = event-data() -> ("VKey"=w1055:T23, "PlatMods"=w1051:T24)  [unwired: 1 in, 2 out]
            n452 = property on="_FontCompression" class="Enum (strict)"() -> ("Key Focus"=w1049:bool)  [unwired: 2 in, 2 out]
            n453 = property on="_MethodIconName" class="Str"() -> ("Key Focus"=w1046:bool)  [unwired: 2 in, 2 out]
            n454 = property on="_TextAlignment" class="Ring (strict)"() -> ("Key Focus"=w1047:bool)  [unwired: 2 in, 2 out]
            n455 = property on="_IconSize" class="Ring (strict)"() -> ("Key Focus"=w1048:bool)  [unwired: 2 in, 2 out]
            n456 = Unbundle By Name(w1058) -> ("Offset.X"=w1053:i32, "Offset.Y"=w1054:i32)
            n457 = Unbundle By Name(w1051) -> ("Ctrl"=w1044:bool)
            n458 = Compound Arithmetic op=AND(invert w1049, invert w1048, invert w1047, invert w1046) -> (w1045:bool)
            n459 = Or(x=w1044, y=w1045) -> (x .or. y?=w1043:bool)
            n460 = case shown="True" w1043 {
              tunnel: w1057 -> [w1060 w1064]
              tunnel: [w1060 w1068] -> w1056
              tunnel: w1055 -> [_ w1067]
              tunnel: w1054 -> [_ w1061]
              tunnel: w1053 -> [_ w1062]
              tunnel: ["Idle" w1066] -> w1052
              tunnel: [_ w1065] -> w1050
              frame False {
              }
              frame True {
                n461 = Bundle By Name(cluster=w1064, "OldOffset.X"=w1062, "OldOffset.Y"=w1061) -> (w1063:T6)
                n462 = case shown="\"Up\"" w1067 {
                  tunnel: w1063 -> [w1075 w1077 w1084 w1091 w1098]
                  tunnel: [w1074 w1077 w1083 w1090 w1097] -> w1068
                  tunnel: w1061 -> [w1073 _ w1082 w1088 w1095]
                  tunnel: w1062 -> [w1071 _ w1080 w1089 w1096]
                  tunnel: ["Generate icon" "Idle" "Generate icon" "Generate icon" "Generate icon"] -> w1066
                  tunnel: [TRUE _ TRUE TRUE TRUE] -> w1065
                  frame "Up" {
                    n463 = Decrement(x=w1073) -> (x-1=w1072:i32)
                    n464 = Bundle By Name(cluster=w1075, "Offset.X"=w1071, "Offset.Y"=w1072) -> (w1074:T6)
                  }
                  frame Default {
                  }
                  frame "Down" {
                    n465 = Increment(x=w1082) -> (x+1=w1081:i32)
                    n466 = Bundle By Name(cluster=w1084, "Offset.X"=w1080, "Offset.Y"=w1081) -> (w1083:T6)
                  }
                  frame "Left" {
                    n467 = Decrement(x=w1089) -> (x-1=w1087:i32)
                    n468 = Bundle By Name(cluster=w1091, "Offset.X"=w1087, "Offset.Y"=w1088) -> (w1090:T6)
                  }
                  frame "Right" {
                    n469 = Increment(x=w1096) -> (x+1=w1094:i32)
                    n470 = Bundle By Name(cluster=w1098, "Offset.X"=w1094, "Offset.Y"=w1095) -> (w1097:T6)
                  }
                }
              }
            }
            n471 = event-data("Discard?"=w1050) -> ()  [unwired: 1 in, 1 out]
          }
          event "_Icons": Value Change {
            (unwired) u16 1 items=["Full", "1 c-term high", "2 c-term high", "3 c-term high"] ("_IconSize")
            n472 = event-data() -> ()  [unwired: 1 in, 1 out]
            n473 = property class="VI"() -> ("Front Panel.WinBounds"=w1113:T8)  [unwired: 2 in, 2 out]
            n474 = Unbundle By Name(w1104) -> ("LayoutChangeExist"=w1102:bool, "StartIconSize"=w1107:u16)
            n475 = local read "_IconSize"() -> (w1111:u16)
            n476 = Equal To 0?(x=w1107) -> (x = 0?=w1108:bool)
            n477 = Equal To 0?(x=w1111) -> (x = 0?=w1112:bool)
            n478 = Select(t=u16 4, s=w1108, f=w1107) -> (s? t:f=w1105:u16)
            n479 = Select(t=u16 4, s=w1112, f=w1111) -> (s? t:f=w1106:u16)
            n480 = Less?(x=w1106, y=w1105) -> (x < y?=w1101:bool)
            n481 = Bundle By Name(cluster=T8 {"Left"=0, "Top"=0, "Right"=500, "Bottom"=0} ("y"), "Right"=w1114) -> (w1115:T8)
            n482 = case shown="True" "_Icons" {
              tunnel: w1114 -> [_ _]
              tunnel: w1115 -> [w1130 w1135]
              tunnel: [w1128 w1134] -> w1118
              tunnel: ["Idle" "UpdateIconFolderList"] -> w1117
              tunnel: w1113 -> [_ w1132]
              frame False {
                n483 = property class="VI"() -> ("Front Panel.WinBounds"=w1131:T8)  [unwired: 2 in, 2 out]
                n484 = Subtract(x=w1131, y=w1130) -> (x-y=w1129:T8)
                n485 = property class="VI"("Front Panel.WinBounds"=w1129) -> (error out=w1128:errorcluster)  [unwired: 2 in, 1 out]
              }
              frame True {
                n486 = Add(x=w1132, y=w1135) -> (x+y=w1136:T8)
                n487 = property class="VI"("Front Panel.WinBounds"=w1136) -> (error out=w1134:errorcluster)  [unwired: 2 in, 1 out]
              }
            }
            n488 = And(x=w1102, y=w1101) -> (x .and. y?=w1100:bool)
            n489 = case shown="True" w1100 {
              tunnel: w1119 -> [_ w1126]
              tunnel: w1118 -> [_ w1125]
              tunnel: "_Icons" -> [_ w1124]
              frame False {
              }
              frame True {
                n490 = Select(t=cluster{"Message":string, "Picture":picture} {"Message"="ShowLeftSide", "Picture"=bytes[0]} ("element"), s=w1124, f=cluster{"Message":string, "Picture":picture} {"Message"="ShowRightSide", "Picture"=bytes[0]} ("element")) -> (s? t:f=w1123:cluster{"Message":string, "Picture":picture})
                n491 = Enqueue Element(queue=w1126, element=w1123, error in (no error)=w1125) -> ()  [unwired: 1 in, 3 out]
              }
            }
            n492 = local write "_IconName"("" ("_IconName")) -> ()
          }
          event "_Folders": Value Change {
            n493 = event-data() -> ()  [unwired: 1 in, 1 out]
          }
          event "_Manage": Value Change {
            n494 = event-data() -> ()  [unwired: 1 in, 1 out]
            n495 = call <resource>:"GDSLvIcon_ManageIconFolderDialog.vi"() -> ("Cancelled"=w1143:bool)  [unwired: 10 in, 1 out]
            n496 = Select(t="Idle", s=w1143, f="UpdateIconFolderList" ("y")) -> (s? t:f=w1142:string)
          }
          event "Icons", "DragIcon": Mouse Move {
            n497 = event-data() -> ("Coords"=w1146:T5)  [unwired: 1 in]
            n498 = Unbundle By Name(w1145) -> ("DraggingIcon"=w1144:bool)
            n499 = case shown="False" w1144 {
              tunnel: w1149 -> [w1162 w1180]
              tunnel: [w1161 w1180] -> w1148
              tunnel: [w1159 "Idle" ("t")] -> w1147
              tunnel: w1146 -> [w1157 _]
              tunnel: w1145 -> [w1154 _]
              frame False {
                n500 = Unbundle By Name(w1154) -> ("IconPos"=w1163:T25)
                n501 = property on="Icons" class="Pict"() -> ("Position"=w1158:T13)  [unwired: 2 in, 2 out]
                n502 = property on="Icons" class="Pict"() -> ("Origin"=w1153:T15)  [unwired: 2 in, 2 out]
                n503 = Subtract(x=w1157, y=w1158) -> (x-y=w1152:T5)
                n504 = Add(x=w1153, y=w1152) -> (x+y=w1151:T5)
                n505 = for {
                  tunnel: w1163 -> [w1173] mode=indexing
                  tunnel: w1151 -> [w1175]
                  tunnel: [w1165] -> w1160
                  tunnel: [w1164] -> w1156
                  i -> [w1164]
                  stop <- w1165 stop-if-true
                  n506 = Unbundle(w1173) -> ("left"=w1172:i16, "top"=w1168:i16, "right"=w1171:i16, "bottom"=w1170:i16)
                  n507 = Unbundle(w1175) -> ("Horizontal"=w1174:i32, "Vertical"=w1169:i32)
                  n508 = In Range and Coerce(upper limit=w1171, x=w1174, lower limit=w1172) -> (In Range?=w1166:bool)  [unwired: 1 out]
                  n509 = In Range and Coerce(upper limit=w1170, x=w1169, lower limit=w1168) -> (In Range?=w1167:bool)  [unwired: 1 out]
                  n510 = And(x=w1166, y=w1167) -> (x .and. y?=w1165:bool)
                }
                n511 = Select(t=w1156, s=w1160, f=-1) -> (s? t:f=w1150:i32)
                n512 = case shown="True" w1160 {
                  tunnel: ["Idle" ("t") "ShowDragIcon" ("t")] -> w1159
                  frame False {
                    n513 = property on="DragIcon" class="Pict"("Visible"=FALSE) -> ()  [unwired: 2 in, 2 out]
                  }
                  frame True {
                  }
                }
                n514 = Bundle By Name(cluster=w1162, "IconSelected"=w1150) -> (w1161:T6)
              }
              frame True {
              }
            }
          }
          event "_IconSearchText": Value Change {
            n515 = event-data() -> ()  [unwired: 1 in, 1 out]
          }
          event Mouse Move {
            n516 = event-data() -> ("Coords"=w1188:T5)  [unwired: 1 in]
            n517 = Unbundle By Name(w1184) -> ("StartTextDraggingPos"=w1183:T5)
            n518 = Unbundle By Name(w1184) -> ("DraggingText"=w1185:bool, "DraggingIcon"=w1187:bool)
            n519 = case shown="True" w1187 {
              tunnel: w1190 -> [w1196 w1219]
              tunnel: [w1195 w1218] -> w1189
              tunnel: w1188 -> [w1192 w1214]
              tunnel: w1184 -> [w1191 _]
              tunnel: [w1194 "UpdateIcon" ("y")] -> w1186
              tunnel: w1185 -> [w1197 _]
              tunnel: w1183 -> [w1193 _]
              frame False {
                n520 = case shown="False" w1197 {
                  tunnel: w1196 -> [w1198 w1212]
                  tunnel: [w1198 w1211] -> w1195
                  tunnel: [_ "Generate icon"] -> w1194
                  tunnel: w1193 -> [_ w1208]
                  tunnel: w1192 -> [_ w1209]
                  tunnel: w1191 -> [_ w1207]
                  frame False {
                  }
                  frame True {
                    n521 = Subtract(x=w1209, y=w1208) -> (x-y=w1204:T5)
                    n522 = Unbundle By Name(w1207) -> ("Offset.X"=w1202:i32, "Offset.Y"=w1201:i32)
                    n523 = Divide(x=w1204, y=u8 4 ("f")) -> (x/y=w1203:cluster{"Horizontal":dbl, "Vertical":dbl})
                    n524 = Unbundle By Name(w1203) -> ("Horizontal"=w1200:dbl, "Vertical"=w1199:dbl)
                    n525 = Bundle By Name(cluster=w1212, "OldOffset.X"=w1202, "OldOffset.Y"=w1201) -> (w1206:T6)
                    n526 = Bundle By Name(cluster=w1206, "Offset.X"=w1200, "Offset.Y"=w1199) -> (w1211:T6)
                  }
                }
              }
              frame True {
                n527 = property on="DragIcon" class="Pict"() -> ("Draw Area Size"=w1224:T7)  [unwired: 2 in, 2 out]
                n528 = property on="_IconPreview" class="Pict"() -> ("Position"=w1222:T13)  [unwired: 2 in, 2 out]
                n529 = Divide(x=w1224, y=2.0 ("Waveform Chart")) -> (x/y=w1225:cluster{"Width":dbl, "Height":dbl})
                n530 = Add(x=w1222, y=T13 {"Left"=0, "Top"=16}) -> (x+y=w1221:T13)
                n531 = Subtract(x=w1214, y=w1225) -> (x-y=w1213:cluster{dbl, dbl})
                n532 = Subtract(x=w1213, y=w1221) -> (x-y=w1216:cluster{dbl, dbl})
                n533 = property on="DragIcon" class="Pict"("Position"=w1213) -> ()  [unwired: 2 in, 2 out]
                n534 = Divide(x=w1216, y=u8 4 ("Disabled")) -> (x/y=w1215:cluster{dbl, dbl})
                n535 = Bundle By Name(cluster=w1219, "BgIconOffset"=w1215) -> (w1218:T6)
              }
            }
          }
          event Mouse Up; Mouse Leave {
            w1227 = FALSE ("DraggingText")
            n536 = event-data() -> ()  [unwired: 1 in, 1 out]
            n537 = Bundle By Name(cluster=w1229, "DraggingText"=w1227) -> (w1228:T6)
            n538 = property on="DragIcon" class="Pict"("Visible"=w1227) -> ()  [unwired: 2 in, 2 out]
          }
          event "_IconPreview": Mouse Up {
            w1232 = FALSE ("Draging")
            n539 = event-data() -> ()  [unwired: 1 in, 3 out]
            n540 = Unbundle By Name(w1231) -> ("IconSelected"=w1230:i32)
            n541 = Bundle By Name(cluster=w1234, "IconDropped"=w1230, "Moving"=w1232, "DraggingIcon"=w1232) -> (w1233:T6)
            n542 = property on="DragIcon" class="Pict"("Visible"=w1232) -> ()  [unwired: 2 in, 2 out]
          }
          event "_IconPreview": Mouse Enter {
            n543 = event-data() -> ()  [unwired: 1 in, 1 out]
            n544 = Unbundle By Name(w1237) -> ("DraggingIcon"=w1235:bool, "IconDropped"=w1236:i32)
            n545 = case shown="True" w1235 {
              tunnel: w1239 -> [w1242 w1243]
              tunnel: [w1241 w1243] -> w1238
              tunnel: w1236 -> [w1240 _]
              frame False {
                n546 = Bundle By Name(cluster=w1242, "IconSelected"=w1240) -> (w1241:T6)
              }
              frame True {
              }
            }
          }
          event "DragIcon": Mouse Down {
            n547 = event-data() -> ("Coords"=w1245:T5)  [unwired: 1 in]
            n548 = property on="DragIcon" class="Pict"() -> ("Draw Area Size"=w1256:T7)  [unwired: 2 in, 2 out]
            n549 = disable-structure shown="Disabled" {
              frame Disabled {
                n550 = call-poly <vilib>:"Set Cursor.vi"("icon"=u16 11) -> ()  [unwired: 9 in, 2 out]
              }
              frame Enabled {
              }
            }
            n551 = Divide(x=w1256, y=2) -> (x/y=w1254:cluster{"Width":dbl, "Height":dbl})
            n552 = property on="_IconPreview" class="Pict"() -> ("Position"=w1252:T13)  [unwired: 2 in, 2 out]
            n553 = Subtract(x=w1245, y=w1254) -> (x-y=w1248:cluster{dbl, dbl})
            n554 = Add(x=w1252, y=T13 {"Left"=0, "Top"=16}) -> (x+y=w1251:T13)
            n555 = Subtract(x=w1248, y=w1251) -> (x-y=w1249:cluster{dbl, dbl})
            n556 = Divide(x=w1249, y=u8 4 ("Disabled")) -> (x/y=w1247:cluster{dbl, dbl})
            n557 = property on="DragIcon" class="Pict"("Position"=w1248, "Visible"=TRUE) -> ()  [unwired: 2 in, 2 out]
            n558 = Bundle By Name(cluster=w1259, "DraggingIcon"=TRUE ("Draging"), "BgIconOffset"=w1247) -> (w1258:T6)
          }
          event "FloodFillMask": Value Change {
            n559 = event-data() -> ()  [unwired: 1 in, 1 out]
            n560 = Unbundle By Name(w1266) -> ("BgIcon"=w1265:u8[][])
            n561 = call <resource>:"GDSIconEditor_CreateImageMask.vi"("Flood Fill"="FloodFillMask", "8-bit pixmap"=w1265) -> ("Array"=w1261:u8[])
            n562 = Bundle By Name(cluster=w1263, "BgIconMask"=w1261) -> (w1262:T6)
          }
          event "_IconPreview": Mouse Down {
            w1271 = 4 ("y")
            # "Check if Mouse down on text, if so Start dragging Text"
            n563 = event-data() -> ("Coords"=w1284:T5)  [unwired: 1 in]
            n564 = property on="_IconPreview" class="Pict"() -> ("Mouse"=w1275:T26)  [unwired: 2 in, 2 out]
            n565 = Unbundle By Name(w1275) -> ("Mouse Position.X"=w1272:i32, "Mouse Position.Y"=w1274:i32)
            n566 = Unbundle By Name(w1268) -> ("IconDropped"=w1283:i32, "TextBounds"=w1282:T22)
            n567 = Unbundle(w1282) -> ("FirstRow"=w1280:i32, "FirstColumn"=w1279:i32, "LastRow"=w1281:i32, "LastColumn"=w1276:i32)
            n568 = Divide(x=w1272, y=w1271) -> (x/y=w1270:dbl)
            n569 = Divide(x=w1274, y=w1271) -> (x/y=w1273:dbl)
            n570 = In Range and Coerce(upper limit=w1281, x=w1273, lower limit=w1280) -> (In Range?=w1278:bool)  [unwired: 1 out]
            n571 = In Range and Coerce(upper limit=w1276, x=w1270, lower limit=w1279) -> (In Range?=w1277:bool)  [unwired: 1 out]
            n572 = And(x=w1278, y=w1277) -> (x .and. y?=w1269:bool)
            n573 = case shown="False" w1269 {
              tunnel: w1287 -> [w1292 w1323]
              tunnel: [w1291 w1320] -> w1286
              tunnel: [w1290 "Idle" ("y")] -> w1285
              tunnel: w1284 -> [w1289 w1314]
              tunnel: w1283 -> [w1288 _]
              tunnel: w1268 -> [_ w1318]
              frame False {
                n574 = case shown="0.." w1288 {
                  selector: w1288 -> [_ w1295]
                  tunnel: w1292 -> [w1294 w1310]
                  tunnel: [w1294 w1309] -> w1291
                  tunnel: ["Idle" ("y") "ShowDragIcon:UpdateIcon" ("y")] -> w1290
                  tunnel: w1289 -> [_ w1296]
                  frame Default {
                  }
                  frame 0.. {
                    n575 = property on="DragIcon" class="Pict"() -> ("Draw Area Size"=w1307:T7)  [unwired: 2 in, 2 out]
                    n576 = Divide(x=w1307, y=2) -> (x/y=w1305:cluster{"Width":dbl, "Height":dbl})
                    n577 = Subtract(x=w1296, y=w1305) -> (x-y=w1299:cluster{dbl, dbl})
                    n578 = property on="_IconPreview" class="Pict"() -> ("Position"=w1303:T13)  [unwired: 2 in, 2 out]
                    n579 = property on="DragIcon" class="Pict"("Position"=w1299) -> ()  [unwired: 2 in, 2 out]
                    n580 = Add(x=w1303, y=T13 {"Left"=0, "Top"=16}) -> (x+y=w1302:T13)
                    n581 = Subtract(x=w1299, y=w1302) -> (x-y=w1300:cluster{dbl, dbl})
                    n582 = Divide(x=w1300, y=u8 4 ("Disabled")) -> (x/y=w1298:cluster{dbl, dbl})
                    n583 = Bundle By Name(cluster=w1310, "IconSelected"=w1295, "DraggingIcon"=TRUE ("Draging"), "BgIconOffset"=w1298) -> (w1309:T6)
                  }
                }
              }
              frame True {
                n584 = Unbundle By Name(w1318) -> ("Offset.X"=w1317:i32, "Offset.Y"=w1316:i32)
                n585 = Bundle("X"=w1317, "Y"=w1316) -> (w1312:cluster{"X":i32, "Y":i32})  [unwired: 1 in]
                n586 = Multiply(x=w1312, y=4) -> (x*y=w1311:cluster{"X":i32, "Y":i32})
                n587 = Subtract(x=w1314, y=w1311) -> (x-y=w1313:T5)
                n588 = Bundle By Name(cluster=w1323, "DraggingIcon"=FALSE, "DraggingText"=TRUE, "StartTextDraggingPos"=w1313) -> (w1320:T6)
              }
            }
          }
          event "DragIcon": Mouse Up {
            w1324 = FALSE ("Draging")
            n589 = event-data() -> ()  [unwired: 1 in, 3 out]
            n590 = Bundle By Name(cluster=w1327, "DraggingIcon"=w1324) -> (w1326:T6)
            n591 = property on="DragIcon" class="Pict"("Visible"=w1324) -> ()  [unwired: 2 in, 2 out]
          }
          event "DragIcon": Mouse Leave {
            n592 = event-data() -> ()  [unwired: 1 in, 1 out]
            n593 = Unbundle By Name(w1330) -> ("DraggingIcon"=w1329:bool)
            n594 = case shown="False" w1329 {
              selector: w1329 -> [w1332 _]
              frame False {
                n595 = property on="DragIcon" class="Pict"("Visible"=w1332) -> ()  [unwired: 2 in, 2 out]
              }
              frame True {
              }
            }
          }
          event "Icons": Mouse Enter {
            n596 = event-data() -> ()  [unwired: 1 in, 1 out]
          }
          event "_IconSize", "_TextAlignment", "_HideHeader": Value Change {
            n597 = event-data() -> ()  [unwired: 1 in, 6 out]
            n598 = Bundle By Name(cluster=w1336, "Offset"=cluster{"X":i32, "Y":i32} {"X"=0, "Y"=0}) -> (w1335:T6)
          }
          event "_OCR": Mouse Enter {
            w1339 = TRUE ("Boolean Text.Font:Bold")
            n599 = event-data() -> ()  [unwired: 1 in, 4 out]
            n600 = property on="_OCR" class="Bool (strict)"("BoolText.FontBold"=w1339, "BoolText.FontUnder"=w1339) -> ()  [unwired: 2 in, 2 out]
          }
          event "_OCR": Mouse Leave {
            w1341 = FALSE ("Boolean Text.Font:Bold")
            n601 = event-data() -> ()  [unwired: 1 in, 4 out]
            n602 = property on="_OCR" class="Bool (strict)"("BoolText.FontBold"=w1341, "BoolText.FontUnder"=w1341) -> ()  [unwired: 2 in, 2 out]
          }
          event "_OCR": Value Change {
            w1344 = FALSE ("Boolean Text.Font:Bold")
            n603 = event-data() -> ()  [unwired: 1 in, 6 out]
            n604 = property on="_OCR" class="Bool (strict)"("BoolText.FontBold"=w1344, "BoolText.FontUnder"=w1344) -> ()  [unwired: 2 in, 2 out]
          }
          event "_FontCompression", "_FontCapitalOnly": Value Change {
            n605 = event-data() -> ()  [unwired: 1 in, 2 out]
          }
          event Value Change {
            n606 = event-data() -> ("OldVal"=w1352:T2)  [unwired: 1 in, 5 out]
            n607 = Unbundle("_BackgroundColor") -> ("Color"=w1347:u32)  [unwired: 1 out]
            n608 = Unbundle(w1352) -> ("Color"=w1350:u32)  [unwired: 1 out]
            n609 = call <resource>:"GDSLvIcon_Convert24bitTo8bitColor.vi"("Color 24bit In"=w1347) -> ("Color out(256)"=w1348:u8)  [unwired: 15 in, 3 out]
            n610 = Unbundle By Name(w1356) -> ("CurrentIcon.ColorsOkayforiconToBeOnTopOf"=w1357:u8[])
            n611 = call <resource>:"GDSLvIcon_Convert24bitTo8bitColor.vi"("Color 24bit In"=w1350) -> ("Color out(256)"=w1349:u8)  [unwired: 15 in, 3 out]
            n612 = Search 1D Array(1D array=w1357, element=w1349) -> (index of element=w1353:i32)  [unwired: 1 in]
            n613 = Replace Array Subset(array=w1357, new element=w1348, index=w1353) -> (w1354:u8[])
            n614 = Bundle By Name(cluster=w1356, "CurrentIcon.ColorsOkayforiconToBeOnTopOf"=w1354) -> (w1355:T6)
          }
          event Value Change {
            n615 = event-data() -> ()  [unwired: 1 in, 6 out]
            n616 = fn#1354() -> (1:w1362:bool)  [unwired: 1 out]
            n617 = Not(x=w1362) -> (.not. x?=w1361:bool)
            n618 = Control Help Window(1:w1361) -> ()  [unwired: 1 in]
          }
          event "_VIPath": Value Change {
            n619 = event-data() -> ()  [unwired: 1 in, 2 out]
            n620 = Unbundle By Name(w1380) -> ("ViRef"=w1379:refnum<vi>)
            n621 = invoke class="VI" method="Save.Instrument"(reference=w1379, "Path to saved file"="_VIPath") -> (reference out=w1376:refnum<vi>, error out=w1364:errorcluster)  [unwired: 4 in, 4 out]
            n622 = call <resource>:"CommonVIs_Wait.vi"("error in"=w1364) -> ("error out"=w1363:errorcluster)  [unwired: 9 in]
            n623 = property class="VI"(reference=w1376, error in=w1363) -> (error out=w1367:errorcluster, "Path"=w1372:path)  [unwired: 1 out]
            n624 = Strip Path(path=w1372) -> (stripped path=w1371:path, name=w1369:string)
            n625 = local write "_VIPath"(w1372) -> ()
            n626 = Unbundle By Name(w1367) -> ("status"=w1374:bool)
            n627 = Select(t=u8 2 ("Disabled"), s=w1367, f=u8 0) -> (s? t:f=w1368:u8)
            n628 = property on="_ApplyHeaderToAll" class="Bool (strict)"("Disabled"=w1368) -> ()  [unwired: 2 in, 2 out]
            n629 = Not(x=w1374) -> (.not. x?=w1373:bool)
            n630 = Bundle By Name(cluster=w1375, "Folder"=w1371, "VI Path"=w1372, "VI name"=w1369, "Icon exist"=w1373) -> (w1370:T6)
          }
          event Timeout {
            n631 = event-data() -> ()  [unwired: 1 in, 3 out]
          }
          event "_TemplateVI": Value Change {
            n632 = event-data() -> ()  [unwired: 1 in, 2 out]
          }
          event Mouse Enter; Mouse Leave {
            n633 = event-data() -> ("CtlRef"=w1394:refnum<vi>, "Type"=w1389:T14)  [unwired: 1 in]
            n634 = property class="Clust (strict)"(reference=w1394) -> (reference out=w1393:refnum<vi>, error out=w1392:errorcluster, "Value"=w1391:T27)  [unwired: 1 in]
            n635 = Equal?(x=w1389, y=lveventtype."Mouse Enter") -> (x = y?=w1387:bool)
            n636 = Bundle By Name(cluster=w1391, "Decal"=w1387) -> (w1390:T27)
            n637 = property class="Clust (strict)"(reference=w1393, error in=w1392, "Value"=w1390) -> ()  [unwired: 2 out]
          }
          event "_EditHeader": Value Change {
            n638 = event-data() -> ()  [unwired: 1 in, 2 out]
            n639 = Unbundle By Name(w1397) -> ("LibraryRef"=w1396:refnum<vi>)
            n640 = Not A Number/Path/Refnum?(number/path/refnum=w1396) -> (NaN/Path/Refnum?=w1395:bool)
            n641 = case shown="False" w1395 {
              tunnel: [w1404 "Edit header"] -> w1399
              frame False {
                w1401 = "Edit VI Header"  # _Edit VI Header
                w1402 = "Edit Library Header"  # _Edit Library Header
                w1403 = "This VI belongs to a library and you can decide if you want to modify the library file's header or just this VI's header."  # _LibraryEditHeaderQuestion
                n642 = Two Button Dialog(message=w1403, 1:w1401, 2:w1402) -> (T button?=w1400:bool)
                n643 = case shown="False" w1400 {
                  tunnel: ["Edit header" "Edit Library Header"] -> w1404
                  frame False {
                  }
                  frame True {
                  }
                }
              }
              frame True {
              }
            }
          }
          event "Accept": Value Change {
            n644 = event-data() -> ()  [unwired: 1 in, 2 out]
          }
          event "_ApplyHeaderToAll": Value Change {
            n645 = event-data() -> ()  [unwired: 1 in, 6 out]
            n646 = Unbundle By Name(w1411) -> ("Text0"=w1410:string)
            n647 = case shown="True" "_ApplyHeaderToAll" {
              tunnel: ["Idle" "UpdateApplyToAllText"] -> w1415
              tunnel: w1410 -> [w1417 _]
              frame False {
                n648 = property on="_ApplyHeaderToAll" class="Bool (strict)"("BoolText.Text"=w1417) -> ()  [unwired: 2 in, 2 out]
              }
              frame True {
              }
            }
            n649 = Bundle By Name(cluster=w1414, "Counter"=0) -> (w1413:T6)
          }
          event "Cancel": Value Change {
            n650 = event-data() -> ()  [unwired: 1 in, 2 out]
          }
          event Panel Close? {
            n651 = event-data() -> ()  [unwired: 1 in, 2 out]
            n652 = event-data("Discard?"=TRUE) -> ()  [unwired: 1 in, 1 out]
          }
        }
      }
      frame "GetImageData" {
        # "Create White mask Color, When Mouse Down"
        n653 = Unbundle By Name(w1434) -> ("Icons"=w1436:T4[], "IconSelected"=w1435:i32)
        n654 = Index Array(array=w1436, index=w1435) -> (element=w1425:T4)
        n655 = call <resource>:"GDSIconEditor_ShrinkImage.vi"("image data"=w1425) -> ("image subset"=w1426:T4)  [unwired: 9 in]
        n656 = call <resource>:"GDSIconEditor_ImageDataTo8Bit.vi"("image data"=w1426) -> ("NoMaskFound"=w1427:bool, "8-bit pixmap"=w1428:u8[][], "mask"=w1432:u8[])  [unwired: 7 in, 1 out]
        n657 = property on="FloodFillMask" class="Bool (strict)"("Visible"=w1427) -> ()  [unwired: 2 in, 2 out]
        n658 = case shown="True" w1427 {
          tunnel: w1428 -> [_ w1441]
          tunnel: w1432 -> [w1438 _]
          tunnel: [w1438 w1440] -> w1429
          frame False {
          }
          frame True {
            n659 = local read "FloodFillMask"() -> (w1439:bool)
            n660 = call <resource>:"GDSIconEditor_CreateImageMask.vi"("Flood Fill"=w1439, "8-bit pixmap"=w1441) -> ("Array"=w1440:u8[])
          }
        }
        n661 = call <vilib>:"Draw Flattened Pixmap.vi"("image data"=w1426) -> ("new picture"=→"DragIcon":picture)  [unwired: 8 in]
        n662 = Bundle By Name(cluster=w1434, "BgIcon"=w1428, "BgIconMask"=w1429) -> (w1433:T6)
      }
      frame "ShowDragIcon", "ShowDragIcon:UpdateIcon" {
        w1474 = 2.0 ("Waveform Chart")
        w1463 = 4 ("x")
        n663 = Unbundle By Name(w1454) -> ("IconNames"=w1446:string[], "Icons"=w1486:T4[], "IconSelected"=w1445:i32, "IconPos"=w1482:T25)
        n664 = Index Array(array=w1446, index=w1445) -> (element=→"_IconName":string)
        n665 = Index Array(array=w1486, index=w1445) -> (element=w1443:T4)
        n666 = Index Array(array=w1482, index=w1445) -> (element=w1481:T28)
        n667 = Unbundle By Name(w1481) -> ("left"=w1480:i16, "top"=w1476:i16, "right"=w1479:i16, "bottom"=w1477:i16)
        n668 = call <resource>:"GDSIconEditor_ShrinkImage.vi"("image data"=w1443) -> ("image subset"=w1442:T4)  [unwired: 9 in]
        n669 = Unbundle By Name(w1442) -> ("Rectangle.right"=w1455:i16, "Rectangle.bottom"=w1456:i16)
        n670 = call <vilib>:"Draw Flattened Pixmap.vi"("image data"=w1442) -> ("new picture"=w1465:picture)  [unwired: 8 in]
        n671 = property on="Icons" class="Pict"() -> ("Position"=w1448:T13)  [unwired: 2 in, 2 out]
        n672 = property on="Icons" class="Pict"() -> ("Origin"=w1449:T15)  [unwired: 2 in, 2 out]
        n673 = Add(x=w1476, y=w1477) -> (x+y=w1475:i16)
        n674 = Add(x=w1480, y=w1479) -> (x+y=w1478:i16)
        n675 = Divide(x=w1475, y=w1474) -> (x/y=w1472:dbl)
        n676 = Divide(x=w1478, y=w1474) -> (x/y=w1473:dbl)
        n677 = Subtract(x=w1448, y=w1449) -> (x-y=w1447:T13)
        n678 = Bundle("right"=w1455, "bottom"=w1456) -> (w1464:cluster{"right":i16, "bottom":i16})  [unwired: 1 in]
        n679 = Bundle(w1473, w1472) -> (w1471:cluster{dbl, dbl})  [unwired: 1 in]
        n680 = Increment(x=w1464) -> (x+1=w1483:cluster{"right":i16, "bottom":i16})
        n681 = Add(x=w1471, y=w1447) -> (x+y=w1470:cluster{dbl, dbl})
        n682 = Divide(x=w1483, y=2.0 ("Waveform Chart")) -> (x/y=w1462:cluster{"right":dbl, "bottom":dbl})
        n683 = Multiply(x=w1463, y=w1462) -> (x*y=w1461:cluster{"right":dbl, "bottom":dbl})
        n684 = Subtract(x=w1470, y=w1461) -> (x-y=w1452:cluster{dbl, dbl})
        n685 = Multiply(x=w1463, y=w1455) -> (x*y=w1467:i32)
        n686 = Multiply(x=w1463, y=w1456) -> (x*y=w1466:i32)
        n687 = Equal?(x=w1450, y="ShowDragIcon:UpdateIcon") -> (x = y?=w1451:bool)
        n688 = Bundle(w1467, w1466) -> (w1468:cluster{i32, i32})  [unwired: 1 in]
        n689 = Select(t="UpdateIcon", s=w1451, f="Idle" ("y")) -> (s? t:f=w1457:string)
        n690 = property on="DragIcon" class="Pict"("Draw Area Size"=w1468, "Value"=w1465, "Visible"=TRUE) -> (error out=w1453:errorcluster)  [unwired: 2 in, 1 out]
        n691 = case shown="False" w1451 {
          tunnel: w1453 -> [w1488 _]
          tunnel: w1452 -> [w1487 _]
          frame False {
            n692 = property on="DragIcon" class="Pict"(error in=w1488, "Position"=w1487) -> ()  [unwired: 1 in, 2 out]
          }
          frame True {
          }
        }
      }
      frame "UpdateIconFolderList" {
        # "C:\\Users\\Mikael\\Documents\\LabVIEW Data\\Glyphs"
        n693 = VI Library() -> (path=w1503:path)
        n694 = call <resource>:"GOOP_GetGDSConfigFolder.vi"() -> ("GDSFolderPath"=w1535:path)
        n695 = call <vilib>:"Set Busy.vi"("error in (no error)"=w1517) -> ("error out"=w1516:errorcluster)  [unwired: 9 in, 1 out]
        n696 = Strip Path(path=w1503) -> (stripped path=w1515:path)  [unwired: 1 out]
        n697 = call <resource>:"GOOP_GetProviderIniFilePath.vi"() -> ("ProviderMainFolder"=w1492:path)  [unwired: 10 in, 1 out]
        n698 = Build Path(base path=w1535, name or relative path="IconFolder.txt") -> (appended path=w1524:path)
        n699 = Read from Text File(file (use dialog)=w1524) -> (text=w1533:string)  [unwired: 3 in, 3 out]
        n700 = Build Path(base path=w1515, name or relative path="resource") -> (appended path=w1504:path)
        n701 = call <vilib>:"Dflt Data Dir.vi"() -> ("App:Default Data Directory"=w1511:path)
        n702 = call <vilib>:"Trim Whitespace.vi"("string"=w1533) -> ("trimmed string"=w1520:string)  [unwired: 1 in]
        n703 = Build Path(base path=w1504, name or relative path="Framework") -> (appended path=w1505:path)
        n704 = Spreadsheet String To Array(delimiter (Tab)="\n", format string="%s", spreadsheet string=w1520, array type (2D Dbl)=string[] []) -> (array=w1498:string[])
        n705 = Build Path(base path=w1511, name or relative path="Glyphs") -> (appended path=w1512:path)
        n706 = Build Path(base path=w1505, name or relative path="Providers") -> (appended path=w1514:path)
        n707 = Build Path(base path=w1514, name or relative path="Icons") -> (appended path=w1500:path)
        n708 = Build Path(base path=w1492, name or relative path="Glyphs") -> (appended path=w1494:path)
        n709 = Build Path(base path=w1492, name or relative path="Icons") -> (appended path=w1491:path)
        n710 = Path To String(path=w1512) -> (string=w1489:string)
        n711 = Path To String(path=w1500) -> (string=w1502:string)
        n712 = Path To String(path=w1494) -> (string=w1501:string)
        n713 = Path To String(path=w1491) -> (string=w1490:string)
        n714 = Build Array(w1502, w1501, w1490, w1489) -> (w1499:string[])
        n715 = Build Array (concatenate)(w1499, w1498) -> (w1497:string[])
        n716 = for {
          tunnel: w1497 -> [w1537] mode=indexing
          tunnel: [w1540] -> w1495 mode=indexing
          tunnel: [w1536] -> w1496 mode=indexing
          n717 = String To Path(string=w1537) -> (path=w1540:path)
          n718 = String Length(string=w1537) -> (length=w1538:i32)
          n719 = Subtract(x=w1538, y=45) -> (x-y=w1539:i32)
          n720 = case shown="1.." w1539 {
            selector: w1539 -> [_ w1549]
            tunnel: w1538 -> [_ _]
            tunnel: w1537 -> [w1542 w1547]
            tunnel: [w1542 w1544] -> w1536
            frame 0, Default {
            }
            frame 1.. {
              n721 = Add(x=w1549, y=3) -> (x+y=w1546:i32)
              n722 = String Subset(string=w1547, offset (0)=w1546) -> (substring=w1545:string)  [unwired: 1 in]
              n723 = Concatenate Strings("..." ("string"), w1545) -> (w1544:string)
            }
          }
        }
        n724 = for {
          tunnel: w1495 -> [w1554] mode=indexing
          shift-right: [w1559] -> w1521
          shift-left: path[] [] -> [w1555]
          shift-right: [w1558] -> w1518
          shift-left: string[] [] -> [w1557]
          tunnel: w1496 -> [w1556] mode=indexing
          n725 = Empty String/Path?(string/path=w1554) -> (empty?=w1552:bool)
          n726 = Search 1D Array(1D array=w1555, element=w1554) -> (index of element=w1553:i32)  [unwired: 1 in]
          n727 = Greater Or Equal To 0?(x=w1553) -> (x >= 0?=w1551:bool)
          n728 = Or(x=w1552, y=w1551) -> (x .or. y?=w1550:bool)
          n729 = case shown="False" w1550 {
            tunnel: w1554 -> [w1563 _]
            tunnel: w1555 -> [w1566 w1576]
            tunnel: [w1565 w1576] -> w1559
            tunnel: w1557 -> [w1561 w1575]
            tunnel: [w1562 w1575] -> w1558
            tunnel: w1556 -> [w1560 _]
            frame False {
              n730 = call <vilib>:"Check if File or Folder Exists.vi"("path"=w1563) -> ("file or folder exists?"=w1564:bool)  [unwired: 8 in, 2 out]
              n731 = case shown="True" w1564 {
                tunnel: w1566 -> [w1568 w1574]
                tunnel: [w1568 w1573] -> w1565
                tunnel: w1563 -> [_ w1572]
                tunnel: w1561 -> [w1567 w1570]
                tunnel: [w1567 w1571] -> w1562
                tunnel: w1560 -> [_ w1569]
                frame False {
                }
                frame True {
                  n732 = Build Array (concatenate)(w1574, w1572) -> (w1573:path[])
                  n733 = Build Array (concatenate)(w1570, w1569) -> (w1571:string[])
                }
              }
            }
            frame True {
            }
          }
        }
        n734 = Build Array (concatenate)("<All icons>" ("y"), w1518) -> (w1528:string[])
        n735 = property on="_Folders" class="Ring (strict)"("Strings []"=w1528, "Value"=1) -> ()  [unwired: 2 in, 2 out]
        n736 = Bundle By Name(cluster=w1527, "Folders"=w1521) -> (w1526:T6)
      }
      frame "PlaceIcon" {
        n737 = Unbundle By Name(w1584) -> ("Icons"=w1586:T4[], "IconSelected"=w1585:i32)
        n738 = Index Array(array=w1586, index=w1585) -> (element=w1578:T4)
        n739 = call <resource>:"GDSIconEditor_ShrinkImage.vi"("image data"=w1578) -> ("image subset"=w1577:T4)  [unwired: 9 in]
        n740 = call <resource>:"GDSIconEditor_ImageDataTo8Bit.vi"("image data"=w1577) -> ("8-bit pixmap"=w1579:u8[][])  [unwired: 7 in, 3 out]
        n741 = Bundle By Name(cluster=w1584, "BgIcon"=w1579, "BgIconOffset"=cluster{"X":i32, "Y":i32} {"X"=0, "Y"=0}) -> (w1583:T6)
      }
      frame "ReadIcons" {
        (unwired) "" ("Name")
        n742 = local read "_Folders"() -> (w1589:u16)
        n743 = Unbundle By Name(w1596) -> ("Folders"=w1595:path[])
        n744 = case shown="0" w1589 {
          tunnel: w1595 -> [w1599 w1604]
          tunnel: w1589 -> [_ w1603]
          tunnel: [w1599 w1600] -> w1594
          frame 0 {
            (unwired) 0 ("index")
          }
          frame Default {
            n745 = Decrement(x=w1603) -> (x-1=w1602:u16)
            n746 = Index Array(array=w1604, index=w1602) -> (element=w1601:path)
            n747 = Build Array(w1601) -> (w1600:path[])
          }
        }
        n748 = call <vilib>:"Set Busy.vi"("error in (no error)"=w1593) -> ("error out"=w1592:errorcluster)  [unwired: 9 in, 1 out]
        n749 = for {
          tunnel: w1594 -> [w1609] mode=indexing
          shift-right: [w1605] -> w1590
          shift-left: cluster{i32, "path out":path}[] [] -> [w1606]
          shift-right: [w1610] -> w1588
          shift-left: w1592 -> [w1607]
          n750 = call <vilib>:"Check if File or Folder Exists.vi"("path"=w1609) -> ("file or folder exists?"=w1608:bool)  [unwired: 8 in, 2 out]
          n751 = case shown="True" w1608 {
            tunnel: [w1612 w1618] -> w1610
            tunnel: w1607 -> [w1612 w1617]
            tunnel: w1609 -> [_ w1616]
            tunnel: w1606 -> [w1611 w1613]
            tunnel: [w1611 w1615] -> w1605
            frame False {
            }
            frame True {
              n752 = call <vilib>:"Recursive File List.vi"("pattern"="*.png", "error in (no error)"=w1617, "Folder Path"=w1616) -> ("error out"=w1620:errorcluster, "All Files in Dir"=w1621:path[])  [unwired: 4 in, 3 out]
              n753 = for {
                tunnel: w1621 -> [w1629] mode=indexing
                tunnel: [w1627] -> w1614 mode=indexing
                shift-right: [w1626] -> w1618
                shift-left: w1620 -> [w1630]
                n754 = File/Directory Info(path=w1629, error in=w1630) -> (path out=w1628:path, size=w1625:i64, error out=w1626:errorcluster)  [unwired: 4 out]
                n755 = Divide(x=w1625, y=i64 100) -> (x/y=w1623:dbl)
                n756 = To Long Integer(number=w1623) -> (32bit integer=w1622:i32)
                n757 = Bundle(w1622, "path out"=w1628) -> (w1627:cluster{i32, "path out":path})  [unwired: 1 in]
              }
              n758 = Build Array (concatenate)(w1613, w1614) -> (w1615:cluster{i32, "path out":path}[])
            }
          }
        }
        n759 = Sort 1D Array(array=w1590) -> (sorted array=w1587:cluster{i32, "path out":path}[])
        n760 = Bundle By Name(cluster=w1596, "IconPaths"=w1587) -> (w1598:T6)
      }
      frame "DrawIcons", "DrawIcons:NoBusy" {
        w1651 = 0  # IconsPerRow
        w1655 = 10  # Border
        w1653 = 15  # Gap
        # "Y"
        # "X"
        n761 = Unbundle By Name(w1644) -> ("IconPaths"=w1636:cluster{i32, "path out":path}[])
        n762 = case shown="\"DrawIcons:NoBusy\"" w1631 {
          tunnel: w1641 -> [w1657 w1659]
          tunnel: [w1657 w1658] -> w1635
          frame "DrawIcons:NoBusy" {
          }
          frame Default {
            n763 = call <vilib>:"Set Busy.vi"("error in (no error)"=w1659) -> ("error out"=w1658:errorcluster)  [unwired: 9 in, 1 out]
          }
        }
        n764 = local read "_IconSearchText"() -> (w1634:string)
        n765 = property on="Icons" class="Pict"() -> ("Draw Area Size"=w1648:T7)  [unwired: 2 in, 2 out]
        n766 = Unbundle By Name(w1648) -> ("Width"=w1654:u32)
        n767 = property on="Icons" class="Pict"("Origin"=T15 {"Horizontal"=0, "Vertical"=0}) -> ()  [unwired: 2 in, 2 out]
        n768 = call <vilib>:"Trim Whitespace.vi"("string"=w1634) -> ("trimmed string"=w1633:string)  [unwired: 1 in]
        n769 = for {
          shift-right: [w1688] -> w1643
          shift-left: w1635 -> [w1671]
          shift-right: [w1675] -> _
          shift-left: w1655 -> [w1683]
          shift-right: [w1686] -> w1638
          shift-left: picture data[5B] ("new picture") -> [w1687]
          shift-right: [w1684] -> w1647
          shift-left: T4[] [] -> [w1685]
          shift-right: [w1676] -> _
          shift-left: w1651 -> [w1677]
          shift-right: [w1674] -> _
          shift-left: w1655 -> [w1678]
          shift-right: [w1679] -> _
          shift-left: TRUE -> [w1682]
          tunnel: w1653 -> [w1681]
          tunnel: w1654 -> [w1680]
          tunnel: w1655 -> [w1673]
          tunnel: w1636 -> [w1672] mode=indexing
          shift-right: [w1670] -> w1645
          shift-left: cluster{i32, i32, i32, i32}[] [] -> [w1669]
          shift-right: [w1667] -> w1639
          shift-left: string[] [] -> [w1668]
          tunnel: w1633 -> [w1666]
          n770 = Unbundle(w1672) -> (w1664:i32, "path out"=w1665:path)
          n771 = case shown="\"\"" w1666 {
            selector: w1666 -> [w1694 _]
            tunnel: w1665 -> [w1695 _]
            tunnel: [w1689 TRUE] -> w1661
            frame Default {
              n772 = To Lower Case(string=w1694) -> (all lower case string=w1691:string)
              n773 = call <vilib>:"Get File Extension.vi"("file"=w1695) -> ("filename without extension"=w1693:string)  [unwired: 6 in, 4 out]
              n774 = To Lower Case(string=w1693) -> (all lower case string=w1692:string)
              n775 = Match Pattern(string=w1692, regular expression=w1691) -> (offset past match=w1690:i32)  [unwired: 1 in, 3 out]
              n776 = Greater Or Equal To 0?(x=w1690) -> (x >= 0?=w1689:bool)
            }
            frame "" {
            }
          }
          n777 = Less Or Equal?(x=w1664, y=50) -> (x <= y?=w1662:bool)
          n778 = And(x=w1661, y=w1662) -> (x .and. y?=w1660:bool)
          n779 = case shown="True" w1660 {
            tunnel: w1665 -> [_ w1709]
            tunnel: w1671 -> [w1705 w1738]
            tunnel: [w1705 w1737] -> w1688
            tunnel: w1687 -> [w1704 w1736]
            tunnel: [w1704 w1715] -> w1686
            tunnel: w1685 -> [w1703 w1721]
            tunnel: [w1703 w1735] -> w1684
            tunnel: w1683 -> [w1701 w1718]
            tunnel: w1682 -> [w1699 w1734]
            tunnel: w1681 -> [_ w1720]
            tunnel: w1680 -> [_ w1731]
            tunnel: [w1699 w1730] -> w1679
            tunnel: w1678 -> [w1700 w1725]
            tunnel: w1677 -> [w1702 w1724]
            tunnel: [w1702 w1723] -> w1676
            tunnel: [w1701 w1713] -> w1675
            tunnel: [w1700 w1717] -> w1674
            tunnel: w1673 -> [_ w1719]
            tunnel: w1669 -> [w1698 w1712]
            tunnel: [w1698 w1711] -> w1670
            tunnel: w1668 -> [w1697 w1707]
            tunnel: [w1697 w1708] -> w1667
            frame False {
            }
            frame True {
              # "Place This Icon on a new row"
              n780 = call <vilib>:"Read PNG File.vi"("error in (no error)"=w1738, "path to PNG file"=w1709) -> ("error out"=w1737:errorcluster, "image data"=w1729:T4)  [unwired: 7 in, 1 out]
              n781 = Unbundle By Name(w1729) -> ("Rectangle"=w1728:T28)
              n782 = Unbundle By Name(w1729) -> ("Rectangle.right"=w1716:i16)
              n783 = Select(t=0, s=w1734, f=w1720) -> (s? t:f=w1733:i32)
              n784 = Add(x=w1733, y=w1718) -> (x+y=w1726:i32)
              n785 = Strip Path(path=w1709) -> (name=w1706:string)  [unwired: 1 out]
              n786 = Add(x=w1726, y=w1716) -> (x+y=w1722:i32)
              n787 = Greater?(x=w1722, y=w1731) -> (0:w1730:bool)
              n788 = Build Array (concatenate)(w1721, w1729) -> (w1735:T4[])
              n789 = case shown="True" w1730 {
                tunnel: [w1743 w1749] -> w1727
                tunnel: w1726 -> [w1740 _]
                tunnel: w1725 -> [w1739 w1744]
                tunnel: w1724 -> [w1742 w1752]
                tunnel: [w1741 1] -> w1723
                tunnel: w1721 -> [_ w1753]
                tunnel: w1720 -> [_ w1747]
                tunnel: w1719 -> [_ w1746]
                tunnel: w1718 -> [_ _]
                tunnel: [w1739 w1745] -> w1717
                tunnel: w1716 -> [_ _]
                frame False {
                  n790 = Bundle(w1740, "Border"=w1739, w1740, "Border"=w1739) -> (w1743:cluster{i32, "Border":i32, i32, "Border":i32})  [unwired: 1 in]
                  n791 = Increment(x=w1742) -> (x+1=w1741:i32)
                }
                frame True {
                  n792 = Delete From Array(array=w1753, length=w1752) -> (deleted portion=w1751:T4[])  [unwired: 1 in, 1 out]
                  n793 = for {
                    tunnel: w1751 -> [w1756] mode=indexing
                    tunnel: [w1755] -> w1750 mode=indexing
                    n794 = Unbundle By Name(w1756) -> ("Rectangle.bottom"=w1755:i16)
                  }
                  n795 = Array Max & Min(array=w1750) -> (max value=w1748:i16)  [unwired: 3 out]
                  n796 = Compound Arithmetic op=ADD(w1744, w1747, w1748) -> (w1745:i32)
                  n797 = Bundle("Border"=w1746, w1745, "Border"=w1746, w1745) -> (w1749:cluster{"Border":i32, i32, "Border":i32, i32})  [unwired: 1 in]
                }
              }
              n798 = Add(x=w1727, y=w1728) -> (x+y=w1710:cluster{i32, i32, i32, i32})
              n799 = Bundle By Name(cluster=w1729, "Rectangle"=w1710) -> (w1714:T4)
              n800 = Build Array (concatenate)(w1712, w1710) -> (w1711:cluster{i32, i32, i32, i32}[])
              n801 = Build Array (concatenate)(w1707, w1706) -> (w1708:string[])
              n802 = Unbundle By Name(w1714) -> ("Rectangle.right"=w1713:i16)
              n803 = call <vilib>:"Draw Flattened Pixmap.vi"("image data"=w1714, "picture"=w1736) -> ("new picture"=w1715:picture)  [unwired: 7 in]
            }
          }
        }
        "Icons" <- w1638
        n804 = property on="DragIcon" class="Pict"("Visible"=FALSE) -> ()  [unwired: 2 in, 2 out]
        n805 = Bundle By Name(cluster=w1644, "Icons"=w1647, "IconPos"=w1645, "IconNames"=w1639) -> (w1656:T6)
        n806 = call <vilib>:"Unset Busy.vi"("error in (no error)"=w1643) -> ()  [unwired: 10 in, 1 out]
      }
      frame "UpdateApplyToAllText" {
        n807 = Unbundle By Name(w1769) -> ("Counter"=w1764:i32, "VIs"=w1761:path[], "Text1"=w1758:string, "Text2"=w1757:string)
        n808 = Increment(x=w1764) -> (x+1=w1768:i32)
        n809 = Bundle By Name(cluster=w1769, "Counter"=w1768) -> (w1762:T6)
        n810 = Array Size(array=w1761) -> (size(s)=w1759:i32)
        n811 = Quotient & Remainder(x=w1764, y=2) -> (x-y*floor(x/y)=w1760:i32)  [unwired: 1 out]
        n812 = case shown="1" w1760 {
          tunnel: [w1771 w1773] -> w1765
          tunnel: w1759 -> [w1772 _]
          tunnel: w1758 -> [_ w1773]
          tunnel: w1757 -> [w1770 _]
          frame 1 {
            n813 = Format Into String(format string=w1770, w1772) -> (resulting string=w1771:string)  [unwired: 2 in, 1 out]
          }
          frame 0, Default {
          }
        }
        n814 = property on="_ApplyHeaderToAll" class="Bool (strict)"("BoolText.Text"=w1765) -> ()  [unwired: 2 in, 2 out]
      }
      frame "Exit" {
        n815 = call <resource>:"GDSError_ClearError.vi"("codes"=i32[] [1052, 8], "error in (no error)"=w1777, "Message popups"=string[] ["Invalid or too long file names!", "File permission error!"]) -> ("error out"=w1774:errorcluster)  [unwired: 15 in, 1 out]
      }
      frame "Edit header" {
        n816 = Unbundle By Name(w1798) -> ("FrameColor"=w1792:u32, "Frame thickness"=w1791:i32, "HeaderIcon"=w1790:u8[][], "Prefix"=w1789:string, "ClassBodyIcon"=w1780:string, "LibraryRef"=w1782:refnum<vi>)
        n817 = Not A Number/Path/Refnum?(number/path/refnum=w1782) -> (NaN/Path/Refnum?=w1783:bool)
        n818 = case shown="False" w1783 {
          tunnel: w1782 -> [w1801 _]
          tunnel: [w1800 enum16{"LvClass", "Library", "X-Control"}."LvClass" ("Type")] -> w1781
          frame False {
            n819 = property class="Library"(reference=w1801) -> ("Path"=w1803:path)  [unwired: 1 in, 2 out]
            n820 = call <vilib>:"Get File Extension.vi"("file"=w1803) -> ("lowercase file extension"=w1802:string)  [unwired: 6 in, 4 out]
            n821 = case shown="\"xctl\"" w1802 {
              tunnel: [enum16{"LvClass", "Library", "X-Control"}."LvClass" ("Type") enum16{"LvClass", "Library", "X-Control"}."Library" ("Type") enum16{"LvClass", "Library", "X-Control"}."X-Control" ("Type")] -> w1800
              frame "lvclass", Default {
              }
              frame "lvlib" {
              }
              frame "xctl" {
              }
            }
          }
          frame True {
          }
        }
        n822 = local read "_BackgroundColor"() -> (w1794:T2)
        n823 = Unbundle By Name(w1794) -> ("Color"=w1793:u32)
        n824 = call <resource>:"GDSIconEditor_HeaderEditorDialog.vi"("BodyBackGround"=w1793, "HeaderText"=w1789, "error in (no error)"=w1796, "HeaderIconIn"=w1790, "Type"=w1781, "FrameThickness(1)"=w1791, "ClassBodyIcon"=w1780, "FrameColor"=w1792) -> ("Cancelled"=w1788:bool, "FrameColorOut"=w1787:u32, "FrameThicknessOut"=w1786:u32, "HeaderIconOut"=w1785:u8[][], "error out"=w1795:errorcluster)  [unwired: 7 in]
        n825 = case shown="False" w1788 {
          tunnel: w1795 -> [w1823 w1829]
          tunnel: [w1823 w1829] -> w1797
          tunnel: ["Generate icon" "Idle"] -> w1784
          tunnel: w1798 -> [w1826 w1827]
          tunnel: [w1825 w1827] -> w1799
          tunnel: w1787 -> [w1821 _]
          tunnel: w1786 -> [w1808 _]
          tunnel: w1785 -> [w1811 _]
          frame False {
            w1820 = u8 32 ("x")
            w1822 = TRUE
            n826 = Array Size(array=w1811) -> (size(s)=w1819:i32[])
            n827 = Index Array(array=w1819) -> (element #1=w1816:i32)  [unwired: 2 in, 1 out]
            n828 = Multiply(x=w1808, y=u8 2) -> (x*y=w1817:u32)
            n829 = Equal To 0?(x=w1816) -> (x = 0?=w1815:bool)
            n830 = Add(x=w1816, y=w1817) -> (x+y=w1813:u32)
            n831 = Increment(x=w1813) -> (x+1=w1814:u32)
            n832 = Select(t=w1813, s=w1815, f=w1814) -> (s? t:f=w1812:u32)
            n833 = Subtract(x=w1820, y=w1812) -> (x-y=w1810:u32)
            n834 = Subtract(x=w1820, y=w1817) -> (x-y=w1809:u32)
            n835 = Bundle By Name(cluster=w1826, "Header exists"=w1822, "Icon exist"=w1822, "FrameColor"=w1821, "Frame thickness"=w1808, "HeaderIcon"=w1811, "BodyIconHeight"=w1810, "BodyIconWidth"=w1809) -> (w1825:T6)
          }
          frame True {
            # "Cancel"
          }
        }
      }
      frame "Edit Library Header" {
        n836 = Unbundle By Name(w1843) -> ("FrameColor"=w1839:u32, "Frame thickness"=w1838:i32, "HeaderIcon"=w1837:u8[][], "Prefix"=w1836:string, "LibraryRef"=w1831:refnum<vi>)
        n837 = disable-structure shown="Enabled" {
          disable-tunnel: w1841 -> [w1856 w1859]
          disable-tunnel: [w1855 w1858] -> w1840
          disable-tunnel: w1839 -> [w1852 _]
          disable-tunnel: w1838 -> [w1851 _]
          disable-tunnel: w1837 -> [w1850 _]
          disable-tunnel: w1836 -> [w1849 _]
          disable-tunnel: [w1848 _] -> _
          disable-tunnel: [w1847 _] -> w1835
          disable-tunnel: [w1846 _] -> w1834
          disable-tunnel: [w1845 _] -> w1833
          disable-tunnel: w1831 -> [_ w1857]
          frame Disabled {
            n838 = local read "_BackgroundColor"() -> (w1854:T2)
            n839 = Unbundle By Name(w1854) -> ("Color"=w1853:u32)
            n840 = call <resource>:"GDSIconEditor_HeaderEditorDialog.vi"("BodyBackGround"=w1853, "HeaderText"=w1849, "error in (no error)"=w1856, "HeaderIconIn"=w1850, "FrameThickness(1)"=w1851, "FrameColor"=w1852) -> ("Cancelled"=w1848:bool, "FrameColorOut"=w1847:u32, "FrameThicknessOut"=w1846:u32, "HeaderIconOut"=w1845:u8[][], "error out"=w1855:errorcluster)  [unwired: 9 in]
          }
          frame Enabled {
            n841 = call <resource>:"GDSLvIcon_DialogUpdateClass.vi"("ClassPath(FilePath/ProjectTreePath/LvCLassRef)"=w1857, "error in (no error)"=w1859) -> ("error out"=w1858:errorcluster)  [unwired: 14 in, 3 out]
          }
        }
        n842 = case shown="True" TRUE {
          tunnel: w1840 -> [w1875 w1881]
          tunnel: [w1875 w1881] -> w1842
          tunnel: ["Generate icon" "Auto find header"] -> w1832
          tunnel: w1843 -> [w1878 w1880]
          tunnel: [w1877 w1880] -> w1844
          tunnel: w1835 -> [w1873 _]
          tunnel: w1834 -> [w1860 _]
          tunnel: w1833 -> [w1863 _]
          frame False {
            w1872 = u8 32 ("x")
            w1874 = TRUE
            n843 = Array Size(array=w1863) -> (size(s)=w1871:i32[])
            n844 = Index Array(array=w1871) -> (element #1=w1868:i32)  [unwired: 2 in, 1 out]
            n845 = Multiply(x=w1860, y=u8 2) -> (x*y=w1869:u32)
            n846 = Equal To 0?(x=w1868) -> (x = 0?=w1867:bool)
            n847 = Add(x=w1868, y=w1869) -> (x+y=w1865:u32)
            n848 = Increment(x=w1865) -> (x+1=w1866:u32)
            n849 = Select(t=w1865, s=w1867, f=w1866) -> (s? t:f=w1864:u32)
            n850 = Subtract(x=w1872, y=w1864) -> (x-y=w1862:u32)
            n851 = Subtract(x=w1872, y=w1869) -> (x-y=w1861:u32)
            n852 = Bundle By Name(cluster=w1878, "Header exists"=w1874, "Icon exist"=w1874, "FrameColor"=w1873, "Frame thickness"=w1860, "HeaderIcon"=w1863, "BodyIconHeight"=w1862, "BodyIconWidth"=w1861) -> (w1877:T6)
          }
          frame True {
            # "Cancel"
          }
        }
      }
      frame "Apply icon" {
        n853 = Unbundle By Name(w1890) -> ("IconOut"=w1901:u8[][], "ViRef"=w1900:refnum<vi>)  [unwired: 2 out]
        n854 = Unbundle By Name(w1890) -> ("StartIconSize"=w1891:u16)
        n855 = local read "_IconSize"() -> (w1883:u16)
        n856 = Reshape Array(w1901, 1024 ("dimension size")) -> (w1896:u8[])
        n857 = Bundle By Name(cluster=T4 {"image type"=0, "image depth"=8, "image"=[], "mask"=[], "colors"=[], "Rectangle"={"left"=0, "top"=0, "right"=32, "bottom"=32}} ("image data"), "image"=w1896) -> (w1897:T4)
        n858 = Not Equal?(x=w1891, y=w1883) -> (x != y?=w1889:bool)
        n859 = invoke class="VI" method="VI Icon.Set from Image Data"(reference=w1900, error in=w1902, "ImageData"=w1897) -> (reference out=w1884:refnum<vi>, error out=w1886:errorcluster)  [unwired: 3 in, 4 out]
        n860 = case shown="True" w1889 {
          tunnel: w1886 -> [w1904 w1909]
          tunnel: [w1904 w1908] -> w1888
          tunnel: w1884 -> [w1903 w1907]
          tunnel: w1883 -> [_ w1906]
          tunnel: [w1903 w1905] -> w1882
          frame False {
          }
          frame True {
            # "We also need to rewire the connector Pane Controls"
            n861 = call <resource>:"GOOP_GetControlRearrangement.vi"("VI Refnum"=w1907, "_IconSize"=w1906, "error in (no error)"=w1909) -> ("ControlsToMove"=w1910:T20, "error out"=w1911:errorcluster)  [unwired: 10 in, 5 out]
            n862 = property class="VI"(reference=w1907, error in=w1911) -> (reference out=w1905:refnum<vi>, error out=w1912:errorcluster, "ConPane"=w1916:refnum<vi>)
            n863 = for {
              tunnel: w1910 -> [w1920] mode=indexing
              tunnel: w1916 -> [w1922]
              shift-right: [w1918] -> w1914
              shift-left: w1912 -> [w1921]
              tunnel: [w1917] -> w1913 mode=indexing
              n864 = Unbundle By Name(w1920) -> ("CtrlRef"=w1917:refnum<vi>, "AfterTerminalIndex"=w1919:i32)
              n865 = invoke class="ConPane" method="AssignCtrlToTerm"(reference=w1922, error in=w1921, "Control"=w1917, "TermIdx"=w1919) -> (error out=w1918:errorcluster)  [unwired: 1 in, 4 out]
            }
            n866 = Close Reference(reference=w1913, error in (no error)=w1914) -> (error out=w1915:errorcluster)
            n867 = Close Reference(reference=w1916, error in (no error)=w1915) -> (error out=w1908:errorcluster)
          }
        }
        n868 = local read "_ApplyHeaderToAll"() -> (w1895:bool)
        n869 = Select(t="ApplyToAll", s=w1895, f="Exit" ("item tag")) -> (s? t:f=w1894:string)
        n870 = call <resource>:"Scripting_SaveVi.vi"("ForceResaving(False)"=TRUE, "error in (no error)"=w1888, "VIRefToSaveIn"=w1882) -> ("error out"=w1887:errorcluster)  [unwired: 7 in, 1 out]
      }
      frame "ApplyToAll" {
        n871 = Unbundle By Name(w1930) -> ("AppRef"=w1923:refnum<vi>, "VIs"=w1931:path[])
        n872 = Unbundle By Name(w1930) -> ("FrameColor"=w1929:u32, "Frame thickness"=w1928:i32, "HeaderIcon"=w1927:u8[][])
        n873 = for {
          tunnel: w1931 -> [w1952] mode=indexing
          tunnel: w1929 -> [w1949]
          tunnel: w1928 -> [w1948]
          tunnel: w1927 -> [w1947]
          shift-right: [w1935] -> w1925
          shift-left: w1926 -> [w1935]
          tunnel: w1923 -> [w1932]
          # "Ignore error since file coudl be read only"
          n874 = call <resource>:"Scripting_OpenViRef.vi"("error in"=w1935, "ViPath/ViName/Viref"=w1952, "AppRef"=w1932) -> ("error out"=w1951:errorcluster, "vi reference"=w1934:refnum<vi>)  [unwired: 6 in, 1 out]
          n875 = call <resource>:"GDSLvIcon_AnalyseViIcon.vi"("ViRef/LvCLassRef/LvLibRef/ViPath/2D_Image"=w1934, "error in (no error)"=w1951) -> ("BodyIcon"=w1946:u8[][], "error out"=w1950:errorcluster)  [unwired: 5 in, 11 out]
          n876 = call <resource>:"GDSLvIcon_CreateIconPicture.vi"("FrameColor"=w1949, "FrameThickness(1)"=w1948, "HeaderIconIn"=w1947, "BodyIconIn"=w1946, "error in (no error)"=w1950) -> ("WholeIconOut"=w1937:u8[][], "error out"=w1936:errorcluster)  [unwired: 9 in, 4 out]
          n877 = Reshape Array(w1937, 1024 ("dimension size")) -> (w1942:u8[])
          n878 = Bundle By Name(cluster=T4 {"image type"=0, "image depth"=8, "image"=[], "mask"=[], "colors"=[], "Rectangle"={"left"=0, "top"=0, "right"=32, "bottom"=32}} ("image data"), "image"=w1942) -> (w1944:T4)
          n879 = invoke class="VI" method="VI Icon.Set from Image Data"(reference=w1934, error in=w1936, "ImageData"=w1944) -> (reference out=w1940:refnum<vi>, error out=w1941:errorcluster)  [unwired: 3 in, 4 out]
          n880 = call <resource>:"Scripting_SaveVi.vi"("ForceResaving(False)"=TRUE, "error in (no error)"=w1941, "VIRefToSaveIn"=w1940) -> ("error out"=w1938:errorcluster, "VIRefToSaveOut"=w1939:refnum<vi>)  [unwired: 7 in]
          n881 = Close Reference(reference=w1939, error in (no error)=w1938) -> ()  [unwired: 1 out]
        }
      }
      frame "Template VI" {
        (unwired) T29."existing file (use LLBs)" ("select mode (2)")
        n882 = File Dialog(6:"*.vi;*.ctl;*.vit;*.ctt;*.llb", 7:"Select template VI" ("prompt")) -> (1:w1961:bool, 2:w1960:bool, 3:w1955:path)  [unwired: 5 in, 1 out]
        n883 = Compound Arithmetic op=AND(w1960, invert w1961) -> (w1959:bool)
        n884 = case shown="True" w1959 {
          tunnel: w1958 -> [w1966 w1970]
          tunnel: [w1966 w1969] -> w1957
          tunnel: ["Idle" w1975] -> w1956
          tunnel: w1955 -> [_ w1971]
          tunnel: w1954 -> [w1964 w1973]
          tunnel: [w1964 w1980] -> w1953
          frame False {
            # "Cancel"
          }
          frame True {
            n885 = Unbundle By Name(w1973) -> ("AppRef"=w1972:refnum<vi>)
            n886 = Open VI Reference(application reference (local)=w1972, vi path=w1971, options=2, error in (no error)=w1970) -> (vi reference=w1967:refnum<vi>, error out=w1969:errorcluster)  [unwired: 2 in]
            n887 = call <resource>:"GDSLvIcon_AnalyseViIcon.vi"("ViRef/LvCLassRef/LvLibRef/ViPath/2D_Image"=w1967, "error in (no error)"=w1969) -> ("FrameColor"=w1978:u32, "FrameThickness(1)"=w1977:u32, "ValidHeaderIcon"=w1979:bool, "HeaderIcon"=w1976:u8[][], "error out"=w1968:errorcluster)  [unwired: 5 in, 8 out]
            n888 = Close Reference(reference=w1967, error in (no error)=w1968) -> ()  [unwired: 1 out]
            n889 = case shown="True" w1979 {
              tunnel: w1973 -> [w1983 w2001]
              tunnel: [w1983 w2000] -> w1980
              tunnel: w1978 -> [_ w1999]
              tunnel: w1977 -> [_ w1986]
              tunnel: w1976 -> [_ w1987]
              tunnel: ["Idle" "Generate icon"] -> w1975
              frame False {
                n890 = One Button Dialog(message="No header found in vi.") -> ()  [unwired: 1 in, 1 out]
              }
              frame True {
                w1996 = u8 32 ("x")
                w1998 = TRUE
                n891 = Array Size(array=w1987) -> (size(s)=w1995:i32[])
                n892 = Index Array(array=w1995) -> (element #1=w1992:i32)  [unwired: 2 in, 1 out]
                n893 = Multiply(x=w1986, y=u8 2) -> (x*y=w1993:u32)
                n894 = Equal To 0?(x=w1992) -> (x = 0?=w1991:bool)
                n895 = Add(x=w1992, y=w1993) -> (x+y=w1989:u32)
                n896 = Increment(x=w1989) -> (x+1=w1990:u32)
                n897 = Select(t=w1989, s=w1991, f=w1990) -> (s? t:f=w1988:u32)
                n898 = Subtract(x=w1996, y=w1988) -> (x-y=w1985:u32)
                n899 = Subtract(x=w1996, y=w1993) -> (x-y=w1984:u32)
                n900 = Bundle By Name(cluster=w2001, "Header exists"=w1998, "Icon exist"=w1998, "FrameColor"=w1999, "Frame thickness"=w1986, "HeaderIcon"=w1987, "BodyIconHeight"=w1985, "BodyIconWidth"=w1984) -> (w2000:T6)
              }
            }
          }
        }
      }
      frame "Error" {
        n901 = call <resource>:"GDSError_LogErrorInformation.vi"("State"=w2004, "LocalVariableData"=w2002, "error in (no error)"=w2003) -> ()  [unwired: 16 in, 1 out]
      }
    }
    n902 = Equal?(x=w64, y="Exit") -> (x = y?=w68:bool)
    n903 = Select(t="Error" ("y"), s=w66, f=w64) -> (s? t:f=w65:string)
  }
  "error out" <- w17
  n904 = property class="VI"("Front Panel.WinBounds"=w26) -> ()  [unwired: 2 in, 2 out]
  n905 = Release Queue(queue=w33) -> ()  [unwired: 2 in, 3 out]
  n906 = Unbundle By Name(w43) -> ("ViRef"=w42:refnum<vi>, "LibraryRef"=w35:refnum<vi>)
  n907 = stacked-sequence {
    tunnel: w17 -> [_]
    frame #0 {
      w2007 = FALSE ("Boolean Text.Font:Bold")
      n908 = property on="_OCR" class="Bool (strict)"("BoolText.FontBold"=w2007, "BoolText.FontUnder"=w2007, "Visible"=FALSE) -> ()  [unwired: 2 in, 2 out]
    }
  }
  n909 = Close Reference(reference=w35) -> (error out=w36:errorcluster)  [unwired: 1 in]
  n910 = case shown="True" w37 {
    tunnel: w42 -> [w2008 w2010]
    tunnel: [w2008 _] -> _
    tunnel: w36 -> [_ _]
    tunnel: [_ FALSE ("Visible")] -> w23
    frame False {
    }
    frame True {
      n911 = Close Reference(reference=w2010) -> ()  [unwired: 1 in, 1 out]
    }
  }
  n912 = property on="DragIcon" class="Pict"("Visible"=w23) -> ()  [unwired: 2 in, 2 out]
